vi "Main PC Station.vi"() -> ()   [LabVIEW 2014]
uses:
  ramki konfiguracyjne.ctl
  CANFrameControl.ctl
  klapki.ctl
  RaptorV_3/Users/K/Desktop/Nowe SbRio/PC/Queue message.ctl
  Program Files (x86)/National Instruments/LabVIEW 2014/examples/Design Patterns/Queued Message Handler/support/QMH Fundamentals - Message Cluster.ctl
  <vilib>/Utility/inputDevices.llb/closeJoystick.vi
  Global GPS.vi
  <vilib>/vision/driver/NI_Vision_Acquisition_Software.lvlib
  <vilib>/ptbypt/NI_PtbyPt.lvlib
panel:
  in  "Zresetuj monitor":bool
  in  "Przestarzała data":bool
  out "czas stopu":timestamp
  out "x-y":dbl
  in  "RESET STM":bool
  in  "STOP ??":bool
  out "timestamp last":timestamp
  out "Waveform Chart":cluster{dbl}(graph)
  in  "Boolean":bool
  out "tim 2":dbl format="%#.8g"
  out "output cluster 3":T1 {"seconds since 1Jan1904" format="%<%H:%M:%S\n%x>T"}
  in  "output cluster 2":T2 {"zadany" format="%<%H:%M:%S\n%x>T"}
  out "output cluster":T3 {"latitude (deg) 2" format="%#.8g"; "longitude (deg) 2" format="%#.8g"}
  out "Numeric 5":i32
  out "wyj pred":cluster{u16, u16, u16, u16, u16, u16} {"?" scale=0.0..65000.0; "?" scale=0.0..65000.0; "?" scale=0.0..65000.0; "?" scale=0.0..65000.0; "?" scale=0.0..65000.0; "?" scale=0.0..65000.0}
  in  "E-Stop":bool
  in  "zerowanie predkosci":T4[](array[typedef])=[{"identifier"=1, "extended?"=FALSE, "type"=0, "payload"=[1, 0, 0, 0, 0, 0, 0, 0]}, {"identifier"=2, "extended?"=FALSE, "type"=0, "payload"=[0, 0, 0, 0, 0, 0, 0]}] {"type" items=["CAN Data", "CAN Remote"]; "identifier" format="%.0x"}
  in  "hamulec 2":T4[](array[typedef])=[{"identifier"=1, "extended?"=FALSE, "type"=0, "payload"=[1, 0, 0, 0, 0, 0, 0, 0]}, {"identifier"=2, "extended?"=FALSE, "type"=0, "payload"=[0, 0, 0, 0, 0, 0, 0]}] {"type" items=["CAN Data", "CAN Remote"]; "identifier" format="%.0x"}
  out "axis info":T5
  out "Digital Waveform Graph":digitalwaveform(graph)
  out "wszystkie":T6(graph)
  out "UDP connection":bool
  in  "Tab Control 2":enum32{"CAN", "FPGA H&S", "SAFETY", "Kamera"}(tab)
  in  "Tab Control":T7(tab)
  in  "STM Prawy ID 2":u32=1
  in  "STM Lewy ID 1":u32=2
  in  "IDD 1":u8=1
  in  "IDD 2":u8=1
  in  "PRZOD L":T8={"Prąd"=10.0, "Kp"=4.0, "Ki"=1.2, "OK Button"=FALSE, "ID"=2, "IDD"=2} {"Ki" format="%.1f"; "Kp" format="%.1f"; "Prąd" format="%.1f"}
  in  "TYL L":T8={"Prąd"=10.0, "Kp"=4.0, "Ki"=1.2, "OK Button"=FALSE, "ID"=2, "IDD"=3} {"Ki" format="%.1f"; "Kp" format="%.1f"; "Prąd" format="%.1f"}
  in  "SRODEK L":T8={"Prąd"=10.0, "Kp"=4.0, "Ki"=1.2000000000000002, "OK Button"=FALSE, "ID"=2, "IDD"=4} {"Ki" format="%.1f"; "Kp" format="%.1f"; "Prąd" format="%.1f"}
  in  "SRODEK P":T8={"Prąd"=10.0, "Kp"=4.0, "Ki"=1.2000000000000002, "OK Button"=FALSE, "ID"=1, "IDD"=3} {"Ki" format="%.1f"; "Kp" format="%.1f"; "Prąd" format="%.1f"}
  in  "TYL P":T8={"Prąd"=10.0, "Kp"=4.0, "Ki"=1.2000000000000002, "OK Button"=FALSE, "ID"=1, "IDD"=4} {"Ki" format="%.1f"; "Kp" format="%.1f"; "Prąd" format="%.1f"}
  in  "PRZOD P":T8={"Prąd"=10.0, "Kp"=4.0000000000000036, "Ki"=1.2000000000000002, "OK Button"=FALSE, "ID"=1, "IDD"=2} {"Ki" format="%.1f"; "Kp" format="%.1f"; "Prąd" format="%.1f"}
  in  "wagi":T9={"l przod"=1.0, "l tyl"=1.0, "l srodek"=1.0, "p przod"=1.0, "p tyl"=1.0, "p srodek"=1.0} {"l przod" format="%#.6g"}
  in  "serwa i pompa":T10={"lewy tyl "=TRUE, "prawy tyl "=TRUE, "lewy przod "=TRUE, "środek"=TRUE, "prawy przod "=TRUE, "serwo 3"=TRUE, "serwo 4 "=TRUE, "przekaznik"=TRUE}
  in  "PWM4":T8={"Prąd"=0.0, "Kp"=4.0, "Ki"=1.2, "OK Button"=FALSE, "ID"=2, "IDD"=2} {"Ki" format="%.1f"; "Kp" format="%.1f"; "Prąd" format="%.1f"}
  in  "PWM5":T8={"Prąd"=0.0, "Kp"=4.0, "Ki"=1.2, "OK Button"=FALSE, "ID"=2, "IDD"=2} {"Ki" format="%.1f"; "Kp" format="%.1f"; "Prąd" format="%.1f"}
  in  "PWM6":T8={"Prąd"=0.0, "Kp"=4.0, "Ki"=1.2, "OK Button"=FALSE, "ID"=2, "IDD"=3} {"Ki" format="%.1f"; "Kp" format="%.1f"; "Prąd" format="%.1f"}
  in  "PWM7":T8={"Prąd"=0.0, "Kp"=4.0, "Ki"=1.2000000000000002, "OK Button"=FALSE, "ID"=2, "IDD"=4} {"Ki" format="%.1f"; "Kp" format="%.1f"; "Prąd" format="%.1f"}
  in  "PWM2":T8={"Prąd"=0.0, "Kp"=4.0, "Ki"=1.2000000000000002, "OK Button"=FALSE, "ID"=1, "IDD"=3} {"Ki" format="%.1f"; "Kp" format="%.1f"; "Prąd" format="%.1f"}
  in  "PWM3":T8={"Prąd"=0.0, "Kp"=4.0, "Ki"=1.2000000000000002, "OK Button"=FALSE, "ID"=1, "IDD"=4} {"Ki" format="%.1f"; "Kp" format="%.1f"; "Prąd" format="%.1f"}
  in  "PWM1":T8={"Prąd"=0.0, "Kp"=4.0000000000000036, "Ki"=1.2000000000000002, "OK Button"=FALSE, "ID"=1, "IDD"=2} {"Ki" format="%.1f"; "Kp" format="%.1f"; "Prąd" format="%.1f"}
  in  "MANIPULATOR ID 3":u32=3
  in  "SERWO 6":u8(slide)=127 scale=0.0..255.0
  in  "SERWO 5":u8(slide)=127 scale=0.0..255.0
  in  "SERWO 4":u8(slide)=127 scale=0.0..255.0
  in  "SERWO 3":u8(slide)=127 scale=0.0..255.0
  in  "Stop głębokość":bool
  in  "Stop wózek":bool
  in  "Wiertło PWM":u8(slide)=128 scale=0.0..255.0
  in  "Wózek PWM":u8(slide)=128 scale=0.0..255.0
  in  "Głębokość PWM":u8(slide)=128 caption="Vertical Pointer Slide" scale=0.0..255.0
  in  "ON/OFF Wiertło":bool
  in  "speed głębokość":u8
  in  "speed wózek":u8
  out "krańcówka 4":bool
  out "krańcówka 3":bool
  out "krańcówka 2":bool
  out "krańcówka":bool
  in  "PROBNK ID 4":u32=3
  in  "Wózek up":bool
  in  "Głębokość down":bool
  in  "Głębokość up":bool
  in  "Wózek down":bool
  out "glebokosc aktualna":dbl(slide) scale=-150.0..220.0
  out "PH":u16(knob) scale=0.0..4095.0
  out "wilgotność i temperatura":string
  out "Środek P":cluster{"mean":dbl, u16}(graph)
  out "PRZOD L":cluster{"mean":dbl, u16}(graph)
  out "TYL L":cluster{"mean":dbl, u16}(graph)
  out "SRODEK L":cluster{"mean":dbl, u16}(graph)
  out "przod P":cluster{"mean":dbl, u16}(graph)
  out "Tyl P":cluster{"mean":dbl, u16}(graph)
  out "Frames":string[][](table)
  in  "Hexadecimal?":bool
  in  "Widocznosc ramek":bool=TRUE
  out "okres 100[ms]":dbl format="%.3g"
  out "ilosc mesagy":dbl
  in  "okres watchdoga":u32=100
  in  "wlacz watchdoga":bool
  out "temperatura":sgl(slide) scale=25.0..70.0
  in  "Total (%)":dbl(knob) scale=0.0..100.0
  in  "System Reset":bool
  out "kolejka odbior":i32
  out "kolejka wysylanie":i32
  in  "stop UDP 2":bool
  in  "udp to sbrio  2":bool
  in  "eventy stop":bool
  out "send ind":i32
  in  "stop queue":bool
  out "receive ind":i32
  in  "UDP odbior in":bool
  in  "stop all":bool
  in  "UDP from sb 2":bool
  in  "UDP to sb 2":bool
  out "eventy ind":i32
  out "Numeric 3":i32
  out "Numeric 4":i32
  out "Image":T11(plugin-control)
  in  "Camera Name":refnum<k21> caption="IMAQdx Session"
  in  "ON/OFF CAM":bool
  out "Acquiring":bool
  in  "Stop 2":bool
  out "Buffer Number 3":u32
  in  "stop UDP":bool
  in  "UDP from sb":bool
  in  "UDP to sb":bool
  out "brak polaczenia":bool
  out "Numeric 2":i32
  out "Numeric":i32
  out "połączenie RT":bool
  out "button 4":bool
  out "button 3":bool
  out "button 2":bool
  out "button 1":bool
  in  "index joya jazda":i32
  in  "device index":i32=4
  out "zakres X":bool
  out "wysylanie":bool
  out "blokadaa":bool
  out "zakres Y":bool
  in  "Sterowanie w ukladzie narzędzia":bool
  out "graph 2":cluster{i32[], i32[]}[](graph)
  out "String wysylany":string
  out "Pz":dbl(slide) scale=0.0..1149.0
  out "Py":dbl(slide) scale=0.0..1075.0
  out "Px":dbl(slide) scale=0.0..1075.0
  out "q5":dbl format="%.2f"
  out "q4":dbl format="%.2f"
  out "q3":dbl format="%.2f"
  out "q2":dbl format="%.2f"
  out "q1":dbl format="%.2f"
  in  "Strin wysłany":string
  out "pwm 1":dbl
  out "pwm 2":dbl
  out "pwm 3":dbl
  out "pwm 4":dbl
  out "pwm 5":dbl
  out "pwm 6":dbl
  out "pwm 7":dbl
  out "zakres Z":bool
  out "cluster manipulator":T12
  in  "UDP odbior":bool
  out "cluster jazda":T13
  out "zak1":bool
  out "zak2":bool
  out "Blokada jazda":bool
  in  "udp to sbrio":bool
  out "hamowanie":bool
  out "hamowaniejazda":dbl
  out "obrotjazda":dbl
  out "skretjazda":dbl
  out "pwmjazda":dbl
  out "obrot":string
  out "skret":string
  out "pwm":string
  out "graph 1":cluster{i32[], i32[]}[](graph)
  out "hamowanie string":string
  out "obrot string":string
  in  "max obrót":dbl(slide) caption="max obrot" scale=0.0..1.0
  in  "max pwm skrecanie":dbl(slide)=1.0 scale=0.0..1.0
  in  "max pwm przod":dbl(slide)=1.0 min=0.0 max=255.0 scale=0.0..1.0
  out "Wysylanie jazda":bool
  out "wyslany":string
  out "jazda":string
  # "STARE"
  # "T-"
  # "T+"
  # "gimbal 1"
  # "gimbal 2"
  # "pochyl chwytak"
  # "PWM 3 os Y\nPWM 4 os X\nPWM 5 T"
  # "chwytak O/Z"
  # "obrot chwytak"
  # "ramie 1"
  # "PWM1 os X \nPWM2 os Y\nPWM 6 T"
  # "ramie 2"
  # "obrot podstawa"
  # "Os Y+"
  # "PWM 7 T"
  # "Os X +"
  # "AKTUALNE"
  # "WYSYLANE"
  # "WYSYLANIE"
  # "- max skrecanie +"
  # "- max jazda +"
  # "hamowanie"
  # "sam OBROT"
  # "- max obrot +"
  # "OBROT"
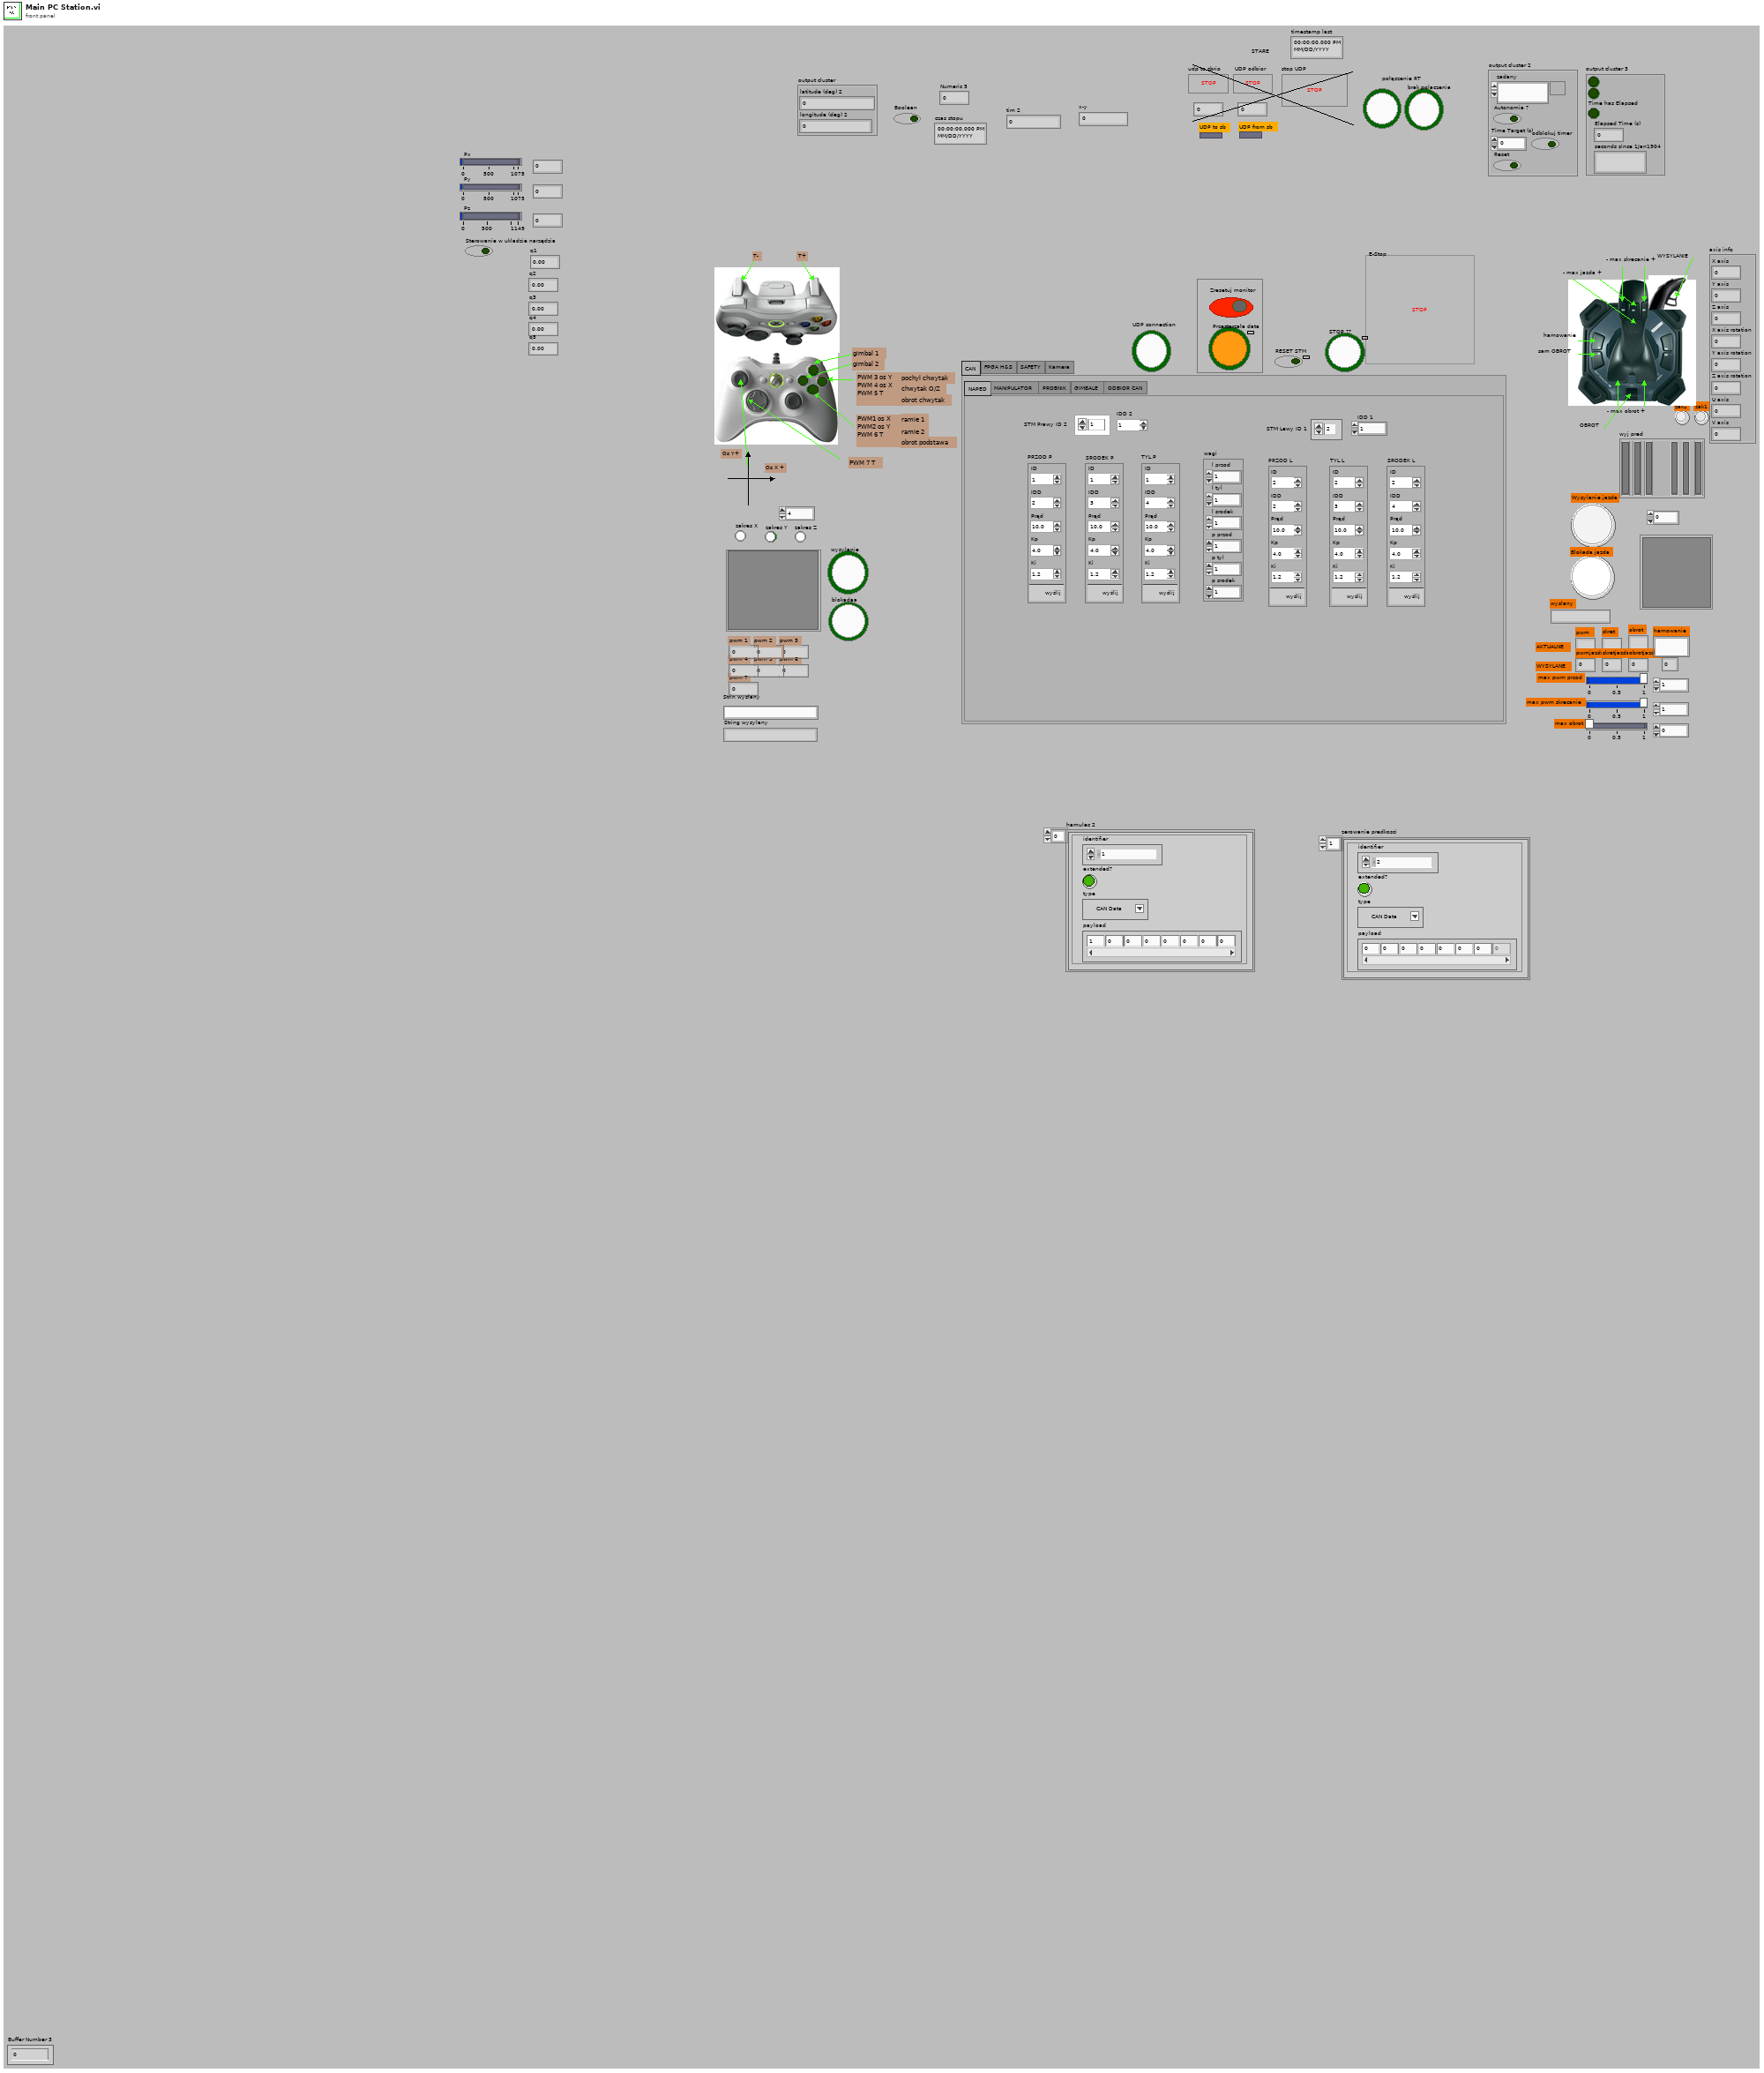
[diagram p1: front panel]
types:
  T1 = cluster{bool, bool, "Time has Elapsed":bool, "Elapsed Time (s)":dbl, "seconds since 1Jan1904":timestamp}
  T2 = cluster{"zadany":timestamp, "Autonomia ?":bool, "Time Target (s)":dbl, "Reset":bool, "odblokuj timer":bool}
  T3 = cluster{"latitude (deg) 2":dbl, "longitude (deg) 2":dbl}
  T4 = typedef "CANFrameControl.ctl" = cluster{"identifier":u32, "extended?":bool, "type":u8, "payload":u8[]}
  T5 = cluster{"X axis":i32, "Y axis":i32, "Z axis":i32, "X axis rotation":i32, "Y axis rotation":i32, "Z axis rotation":i32, "U axis":i32, "V axis":i32}
  T6 = cluster{"mean":dbl, "mean":dbl, "mean":dbl, "mean":dbl, "mean":dbl, "mean":dbl}
  T7 = enum32{"NAPED", "MANIPULATOR", "PROBNIK", "GIMBALE", "ODBIOR CAN"}
  T8 = typedef "ramki konfiguracyjne.ctl" = cluster{"Prąd":dbl, "Kp":dbl, "Ki":dbl, "OK Button":bool, "ID":u32, "IDD":u8}
  T9 = cluster{"l przod":dbl, "l tyl":dbl, "l srodek":dbl, "p przod":dbl, "p tyl":dbl, "p srodek":dbl}
  T10 = typedef "klapki.ctl" = cluster{"lewy tyl ":bool, "prawy tyl ":bool, "lewy przod ":bool, "środek":bool, "prawy przod ":bool, "serwo 3":bool, "serwo 4 ":bool, "przekaznik":bool}
  T11 = typedef "IMAQ Image.ctl" = refnum<image>
  T12 = cluster{"pwm 1":dbl, "pwm 2":dbl, "pwm 3":dbl, "pwm 4":dbl, "pwm 5":dbl, "pwm 6":dbl, "pwm 7":dbl}
  T13 = cluster{"pwmjazda":dbl, "skretjazda":dbl, "obrotjazda":dbl, "hamowaniejazda":dbl}
  T14 = typedef "QMH Fundamentals - Message Cluster.ctl" = cluster{"Message":string, "Message Data":variant}
  T15 = typedef "Queue message.ctl" = cluster{"Message":string, "Message Data":variant}
  T16 = enum16{"Rising Edge", "Falling Edge", "Any Edge"}
  T17 = typedef "Wyjscia joya.ctl" = cluster{"button 1":bool, "button 2":bool, "button 3":bool, "button 4":bool, "button 5":bool, "button 6":bool, "button 7":bool, "button 8":bool, "button 9":bool, "POV":bool, "button 10":bool}
  T18 = cluster{"STM Lewy ID 1":u32, "STM Prawy ID 2":u32, "IDD 1":u8, "IDD 2":u8}
  T19 = cluster{"remote port":u16, u32, "port":refnum<k16>, "error out":errorcluster}
  T20 = cluster{"cluster_jazda":cluster{"pwmjazda":dbl, "skretjazda":dbl, "obrotjazda":dbl, "hamowaniejazda":dbl}, "cluster_manipulator":cluster{"pwm 1":dbl, "pwm 2":dbl, "pwm 3":dbl, "pwm 4":dbl, "pwm 5":dbl, "pwm 6":dbl, "pwm 7":dbl}, "GIMBALE":cluster{"Gimbal 1":cluster{"OSY":dbl, "OSY X":dbl}, "Gimbal 2":cluster{"OSY":dbl, "OSY X":dbl}}}
  T21 = cluster{"button 1":bool, "button 2":bool, "button 3":bool, "button 4":bool, "button 5":bool}
  T22 = typedef "IMAQdx.ctl" = refnum<k21>
  T23 = cluster{"SERWO 6":u8, "SERWO 5":u8, "SERWO 4":u8, "SERWO 3":u8, "ON/OFF Wiertło":bool, "Wiertło PWM":u8, "Wózek PWM":u8, "Stop głębokość":bool, "Głębokość PWM":u8, "speed wózek":u8, "Wózek up":bool, "Wózek down":bool, "Stop wózek":bool, "PROBNK ID 4":u32}
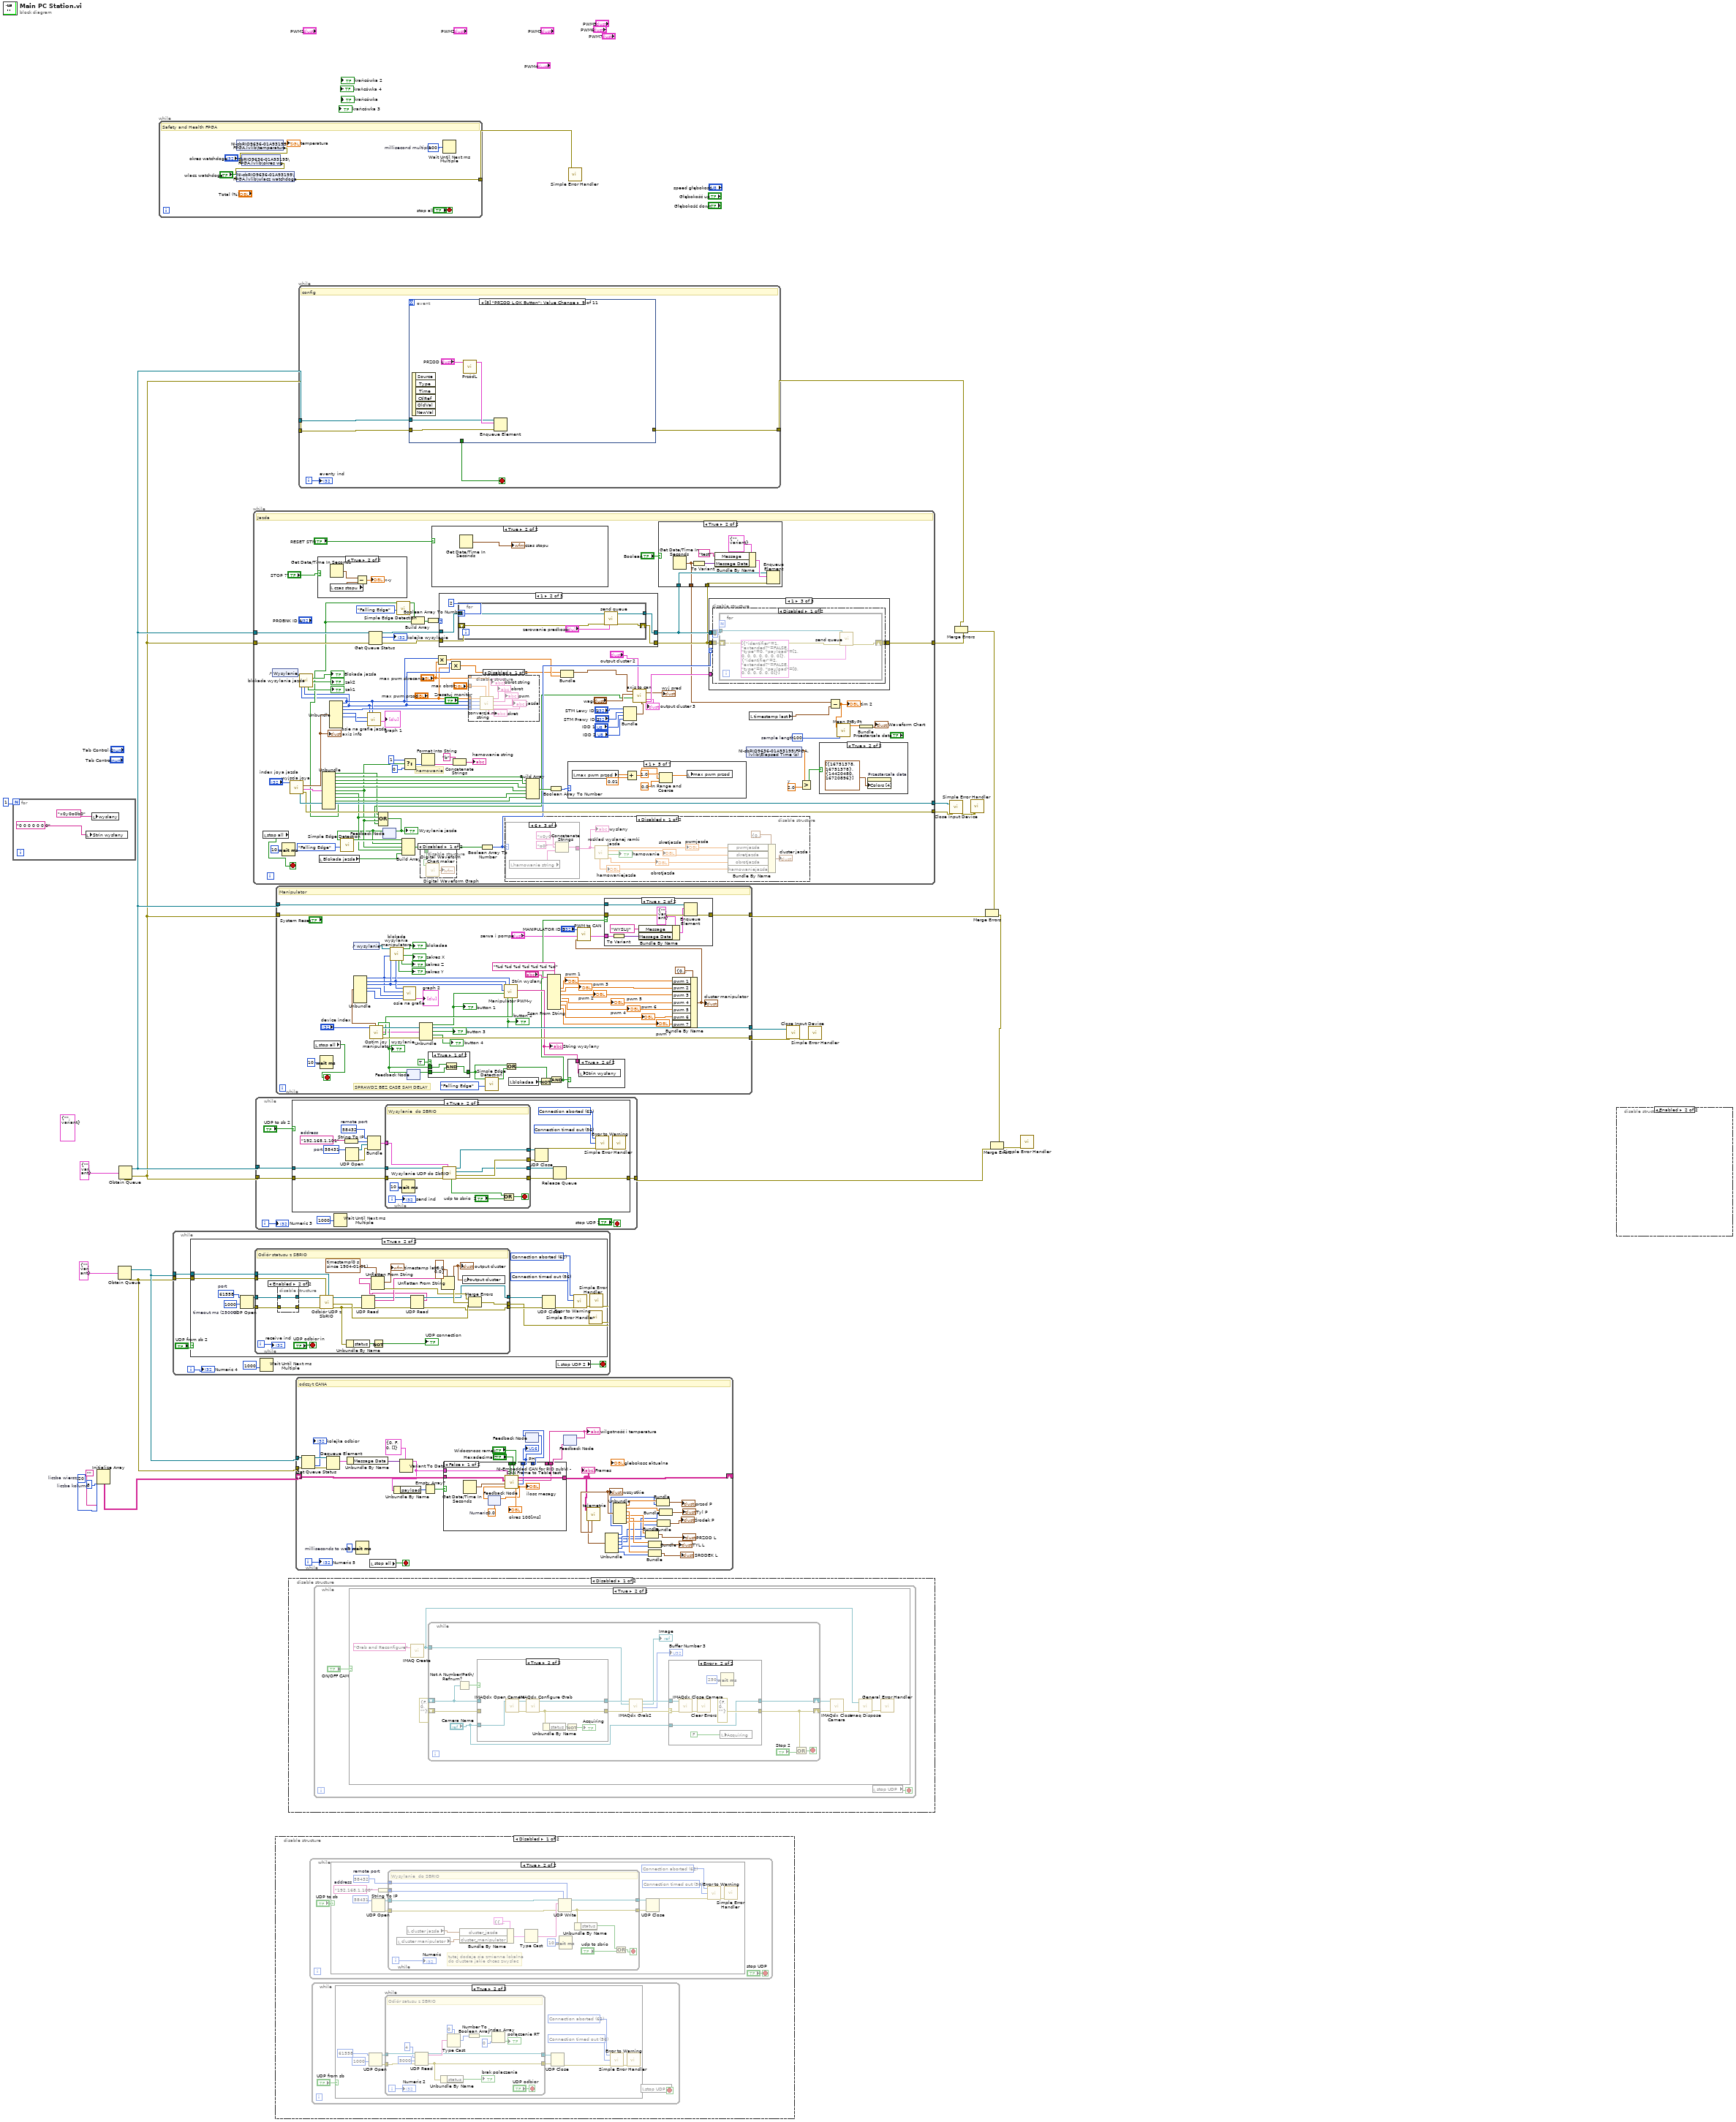
[diagram p0: block diagram]
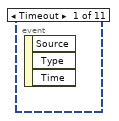
[diagram p7: hidden frame]
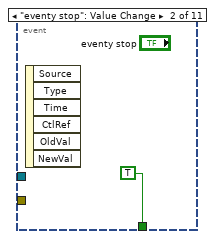
[diagram p8: hidden frame]
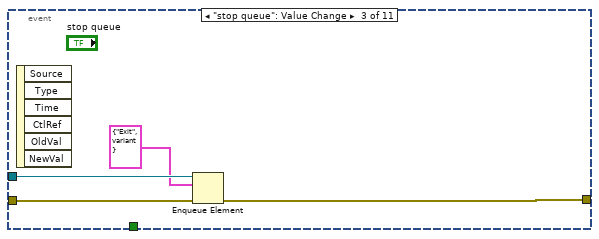
[diagram p9: hidden frame]
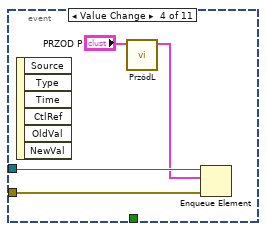
[diagram p10: hidden frame]
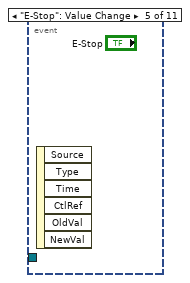
[diagram p11: hidden frame]
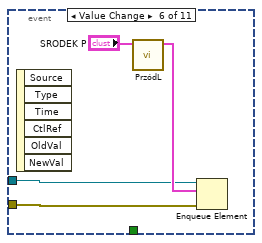
[diagram p12: hidden frame]
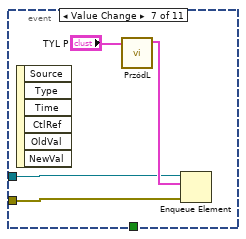
[diagram p13: hidden frame]
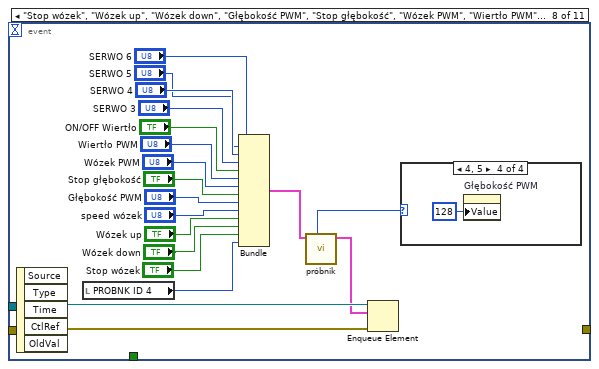
[diagram p14: hidden frame]
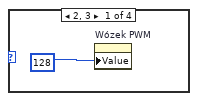
[diagram p15: hidden frame]
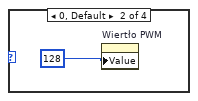
[diagram p16: hidden frame]
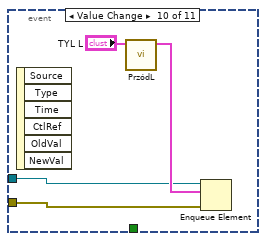
[diagram p18: hidden frame]
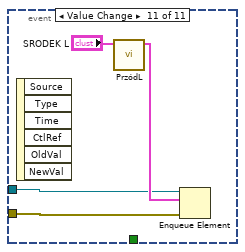
[diagram p19: hidden frame]
diagram:
  w8 = 20  # liczba wierszy
  w7 = 5  # liczba kolumn
  (unwired) T15 {"Message"="", "Message Data"=variant} ("Message Cluster")
  n1 = for {
    N: 1 -> [_]
    n2 = local write "Strin wysłany"("0 0 0 0 0 0 0") -> ()
    n3 = local write "wyslany"("x0y0o0b0") -> ()
  }
  n4 = Initialize Array("" ("Empty String Constant"), w8, w7) -> (w5:string[][])
  n5 = Obtain Queue(element data type=T14 {"Message"="", "Message Data"=variant} ("Message Cluster")) -> (queue out=w3:refnum<queue>, error out=w2:errorcluster)  [unwired: 4 in, 1 out]
  n6 = Obtain Queue(element data type=T14 {"Message"="", "Message Data"=variant} ("Message Cluster")) -> (queue out=w13:refnum<queue>, error out=w12:errorcluster)  [unwired: 4 in, 1 out]
  n7 = while {
    tunnel: [w30] -> w1
    stop <- "stop all" stop-if-true
    w34 = u32 100  # millisecond multiple
    # "Safety and Health FPGA"
    n8 = shared-variable "NI-sbRIO9636-01A93195\\FPGA.lvlib\\temperatura"() -> (→"temperatura":sgl, error out=w29:errorcluster)  [unwired: 1 in]
    n9 = shared-variable "NI-sbRIO9636-01A93195\\FPGA.lvlib\\okres wg"("okres watchdoga", error in=w29) -> (error out=w31:errorcluster)
    n10 = shared-variable "NI-sbRIO9636-01A93195\\FPGA.lvlib\\wlacz watchdoga"("wlacz watchdoga", error in=w31) -> (error out=w30:errorcluster)
    n11 = Wait Until Next ms Multiple(millisecond multiple=w34) -> ()  [unwired: 1 out]
  }
  n12 = while {
    tunnel: w3 -> [w37]
    tunnel: w2 -> [w36]
    i -> [w39]
    stop <- w40 stop-if-true
    n13 = case shown="True" "UDP from sb 2" {
      tunnel: w37 -> [_ w44]
      tunnel: w36 -> [_ w43]
      frame False {
      }
      frame True {
        w53 = 1000  # timeout ms (25000)
        w50 = 56 items=["No Error", "Argument Error", "Memory Full", "Out of Zone", "End of File", "File Already Open", "Generic File IO Error", "File Not Found", "File Permission Error", "Disk Full", "Duplicate Path", "Too Many Files Open", "Not Enabled", "Resource File Not Found", "Cannot Add Resource", "Resource Not Found", "Image Not Found", "Image Memory Error", "Pen Does Not Exist", "Config Bad Type", "Config Token Not Found", "Config Parse Error", "Config Memory Error", "Bad External Code Format", "Bad External Code Offset", "External Code Not Present", "Null Window", "Destroy Window Mixup", "Null Menu", "Print Aborted", "Bad Print Record", "Print Driver Error", "Windows Error During Print", "Memory Error During Print", "Print Dialog Error", "Generic Print Error", "Invalid Device Refnum", "Device Not Found", "Device Parameter Error", "Device Unit Error", "Can't Open Device", "Device Call Aborted", "Generic Error", "Cancelled By User", "Object ID Too Low", "Object ID Too High", "Object Not In Heap", "Unknown Heap", "Bad DefProc ID", "DefProc Not In Table", "Message Out Of Range", "Null Method", "Unknown Message", "Manager Call Not Supported", "Bad address", "Connection In progress", "Connection timed out", "Connection is already in progress", "Network attribute not supported", "Network error", "Address in use", "System out of memory", "Connection aborted", "Connection refused", "Connection is not connected", "Connection is already connected", "Connection closed", "Initialize error (interapplication manager)", "Bad occurrence", "Wait on unbound occurrence handler", "Occurrence queue overflow", "Bad path", "Semaphore not signaled", "Unrecognized type (interapplication manager)"] ("3rd Error to Convert")
        w51 = 62 items=["No Error", "Argument Error", "Memory Full", "Out of Zone", "End of File", "File Already Open", "Generic File IO Error", "File Not Found", "File Permission Error", "Disk Full", "Duplicate Path", "Too Many Files Open", "Not Enabled", "Resource File Not Found", "Cannot Add Resource", "Resource Not Found", "Image Not Found", "Image Memory Error", "Pen Does Not Exist", "Config Bad Type", "Config Token Not Found", "Config Parse Error", "Config Memory Error", "Bad External Code Format", "Bad External Code Offset", "External Code Not Present", "Null Window", "Destroy Window Mixup", "Null Menu", "Print Aborted", "Bad Print Record", "Print Driver Error", "Windows Error During Print", "Memory Error During Print", "Print Dialog Error", "Generic Print Error", "Invalid Device Refnum", "Device Not Found", "Device Parameter Error", "Device Unit Error", "Can't Open Device", "Device Call Aborted", "Generic Error", "Cancelled By User", "Object ID Too Low", "Object ID Too High", "Object Not In Heap", "Unknown Heap", "Bad DefProc ID", "DefProc Not In Table", "Message Out Of Range", "Null Method", "Unknown Message", "Manager Call Not Supported", "Bad address", "Connection In progress", "Connection timed out", "Connection is already in progress", "Network attribute not supported", "Network error", "Address in use", "System out of memory", "Connection aborted", "Connection refused", "Connection is not connected", "Connection is already connected", "Connection closed", "Initialize error (interapplication manager)", "Bad occurrence", "Wait on unbound occurrence handler", "Occurrence queue overflow", "Bad path", "Semaphore not signaled", "Unrecognized type (interapplication manager)"] ("1st Error to Convert")
        w45 = u16 61558  # port
        n14 = UDP Open(9:w53, 11:w45) -> (port=w46:refnum<k16>, 0:w47:errorcluster)  [unwired: 3 in, 1 out]
        n15 = while {
          tunnel: w46 -> [w64]
          tunnel: w47 -> [w65]
          tunnel: [w56] -> w48
          tunnel: [w59] -> w54
          tunnel: [w71] -> w42
          tunnel: w44 -> [w76]
          tunnel: w43 -> [w75]
          i -> [w78]
          stop <- "UDP odbior in" stop-if-true
          # "Odiór statusu z SBRIO"
          n16 = disable-structure shown="Enabled" {
            disable-tunnel: w65 -> [w84 w85]
            disable-tunnel: w64 -> [w83 w86]
            disable-tunnel: [w82 w86] -> w63
            disable-tunnel: [w81 w85] -> w62
            frame Disabled {
              n17 = UDP Read(connection ID=w83, 8:w84) -> (error out=w81:errorcluster, 3:w82:refnum<k16>)  [unwired: 2 in, 3 out]
            }
            frame Enabled {
            }
          }
          n18 = call "Odbiór UDP z SbRIO.vi"("Queue in"=w76, "error in queue"=w75, "error in udp (no error)"=w62, "port"=w63) -> ("error out udp"=w69:errorcluster, "error out variant"=w72:errorcluster, "UDP Network Connection out"=w67:refnum<k16>)  [unwired: 5 in]
          n19 = Unbundle By Name(w69) -> ("status"=w79:bool)
          n20 = UDP Read(connection ID=w67, 8:w69) -> (data out=w66:string, error out=w58:errorcluster, 3:w57:refnum<k16>)  [unwired: 2 in, 2 out]
          n21 = Not(x=w79) -> (.not. x?=→"UDP connection":bool)
          n22 = UDP Read(connection ID=w57, 8:w58) -> (data out=w55:string, error out=w59:errorcluster, 3:w56:refnum<k16>)  [unwired: 2 in, 2 out]
          n23 = Unflatten From String(type=timestamp(0 s since 1904-01-01) ("seconds since 1Jan1904"), binary string=w55) -> (value=→"timestamp last":timestamp, error out=w68:errorcluster)  [unwired: 3 in, 1 out]
          n24 = Unflatten From String(type=T3 {"latitude (deg) 2"=0.0, "longitude (deg) 2"=0.0} ("output cluster"), binary string=w66) -> (value=w70:T3, error out=w73:errorcluster)  [unwired: 3 in, 1 out]
          "output cluster" <- w70
          n25 = global write "Global GPS.vi" "output cluster"(w70) -> ()
          n26 = Merge Errors(w68, w73, w72) -> (w71:errorcluster)
          "receive ind" <- w78
        }
        n27 = UDP Close(connection ID=w48, 8:w54) -> (error out=w52:errorcluster)  [unwired: 1 out]
        n28 = call <vilib>:"Error to Warning.vi"("1st Error to Convert"=w51, "3rd Error to Convert"=w50, "error in"=w52) -> ("warning out"=w49:errorcluster)  [unwired: 3 in, 9 out]
        n29 = call <vilib>:"Simple Error Handler.vi"("error in (no error)"=w42) -> ()  [unwired: 1 in, 8 out]
        n30 = call <vilib>:"Simple Error Handler.vi"("error in (no error)"=w49) -> ()  [unwired: 1 in, 8 out]
      }
    }
    n31 = Wait Until Next ms Multiple(millisecond multiple=u32 1000 ("milliseconds to wait")) -> ()  [unwired: 1 out]
    n32 = local read "stop UDP 2"() -> (w40:bool)
    "Numeric 4" <- w39
  }
  n33 = while {
    tunnel: [w155] -> w24
    tunnel: [w154] -> w23
    tunnel: w13 -> [w134]
    tunnel: w12 -> [w135]
    tunnel: [w136] -> w14
    stop <- w127 stop-if-true
    w89 = 2.0  # y
    w93 = 100  # sample length
    # "hamowanie"
    # "Jazda"
    n34 = local read "stop all"() -> (w127:bool)
    n35 = control-ref of="Wysylanie jazda"() -> (w167:refnum<vi>)
    n36 = Wait (ms)(milliseconds to wait=u32 10) -> ()  [unwired: 1 out]
    n37 = call "wyjscia joya.vi"("index joya jazda"="index joya jazda") -> ("error out"=w154:errorcluster, "wyjscia joya"=w153:T17, "axis info"=w124:T5, "Refnum out"=w155:refnum<k1>)  [unwired: 5 in]
    "axis info" <- w124
    n38 = case shown="True" "STOP ??" {
      frame False {
      }
      frame True {
        n39 = Get Date/Time In Seconds() -> (seconds since 1Jan1904=w172:timestamp)
        n40 = local read "czas stopu"() -> (w171:timestamp)
        n41 = Subtract(x=w172, y=w171) -> (x-y=→"x-y":dbl)
      }
    }
    n42 = local read "Blokada jazda"() -> (w168:bool)
    n43 = Unbundle(w153) -> ("button 1"=w146:bool, "button 2"=w152:bool, "button 3"=w151:bool, "button 4"=w150:bool, "button 5"=w149:bool, "button 6"=w144:bool, "button 7"=w145:bool, "button 8"=w148:bool, "button 9"=w147:bool, "POV"=w121:bool)  [unwired: 1 out]
    n44 = Unbundle(w124) -> ("X axis"=w110:i32, "Y axis"=w107:i32, "Z axis"=w138:i32, "X axis rotation"=w139:i32, "Y axis rotation"=w140:i32)  [unwired: 3 out]
    n45 = call "blokada wysylania jazda.vi"("Y axis"=w107, "X axis"=w110, "Boolean in"=w167) -> ("zak2"=→"zak2":bool, "blokada jazdy"=→"Blokada jazda":bool, "zak1"=→"zak1":bool)  [unwired: 6 in]
    n46 = call "osie na grafie jazda.vi"("Y axis rotation"=w140, "X axis rotation"=w139, "Y axis"=w107, "X axis"=w110) -> ("graph 1"=→"graph 1":cluster{i32[], i32[]}[])  [unwired: 7 in]
    n47 = Get Queue Status(queue=w134, error in (no error)=w135) -> (queue out=w126:refnum<queue>, error out=w125:errorcluster, # elements in queue=→"kolejka wysylanie":i32)  [unwired: 1 in, 5 out]
    n48 = feedback #1() -> (w130:bool)  [unwired: 1 in]
    n49 = call "Simple Edge Detection.vi"("Mode"=T16."Falling Edge", "clk_in"=w130) -> ("edge?"=w157:bool)  [unwired: 9 in]
    n50 = call "Simple Edge Detection.vi"("Mode"=T16."Falling Edge", "clk_in"=w121) -> ("edge?"=w122:bool)  [unwired: 9 in]
    n51 = Build Array(w157, w130, w144, w145, w168) -> (w129:bool[])
    n52 = Select(t=1, s=w144, f=0) -> (s? t:f=w143:i32)
    n53 = Build Array(w122, w121) -> (w120:bool[])
    n54 = disable-structure shown="Disabled" {
      disable-tunnel: w129 -> [w233 _]
      frame Disabled {
        n55 = call "Digital Waveform Chart maker.vi"("Array"=w233) -> ("digital waveform"=→"Digital Waveform Graph":digitalwaveform)  [unwired: 3 in]
      }
      frame Enabled {
      }
    }
    n56 = Format Into String(w143) -> (resulting string=w161:string)  [unwired: 3 in, 1 out]
    n57 = Boolean Array To Number(Boolean array=w120) -> (number=w119:u32)
    n58 = case shown="True" "RESET STM" {
      frame False {
      }
      frame True {
        n59 = Get Date/Time In Seconds() -> (seconds since 1Jan1904=→"czas stopu":timestamp)
      }
    }
    n60 = Multiply(x=w110, y="max pwm skrecanie") -> (x*y=w109:dbl)
    n61 = case shown="1" w119 {
      tunnel: [w216 w218 w228] -> w100
      tunnel: w126 -> [w216 w221 w229]
      tunnel: w125 -> [w215 w220 w230]
      tunnel: [w215 w219 w231] -> w99
      frame 0, Default {
      }
      frame 1 {
        n62 = for {
          N: 2 -> [_]
          tunnel: w221 -> [w226]
          shift-right: [w224] -> w219
          shift-left: w220 -> [w225]
          tunnel: [w222] -> w218
          n63 = call "send queue.vi"("zerowanie predkosci"="zerowanie predkosci", "error in (no error)"=w225, "Queue in"=w226) -> ("error out"=w224:errorcluster, "queue out"=w222:refnum<queue>)  [unwired: 7 in]
        }
      }
      frame 2 {
        n64 = call "send queue.vi"("zerowanie predkosci"="hamulec 2", "error in (no error)"=w230, "Queue in"=w229) -> ("error out"=w231:errorcluster, "queue out"=w228:refnum<queue>)  [unwired: 7 in]
      }
    }
    n65 = Multiply(x=w107, y="max pwm przod") -> (x*y=w108:dbl)
    n66 = Concatenate Strings("b", w161) -> (→"hamowanie string":string)
    n67 = disable-structure shown="Disabled" {
      disable-tunnel: w138 -> [w192 _]
      disable-tunnel: w107 -> [w191 _]
      disable-tunnel: w110 -> [w190 _]
      disable-tunnel: "max obrót" -> [w188 _]
      disable-tunnel: "max pwm przod" -> [w184 _]
      disable-tunnel: "max pwm skrecanie" -> [w182 _]
      frame Disabled {
        n68 = call "conversja na string.vi"("max pwm skrecanie"=w182, "max obrót"=w188, "Z axis"=w192, "Y axis"=w191, "X axis"=w190, "max pwm przod"=w184) -> ("String 5"=→"jazda":string, "String 3"=→"pwm":string, "String 2"=→"obrot":string, "String 4"=→"obrot string":string, "String"=→"skret":string)  [unwired: 1 in]
      }
      frame Enabled {
      }
    }
    n69 = Boolean Array To Number(Boolean array=w129) -> (number=w128:u32)
    n70 = disable-structure shown="Disabled" {
      disable-tunnel: w128 -> [w193 _]
      frame Disabled {
        n71 = case shown="6" w193 {
          tunnel: ["x0y0o0b0" w205 w209 w214] -> w198
          frame 1, Default {
          }
          frame 2 {
            n72 = local read "jazda"() -> (w206:string)
            n73 = Concatenate Strings(w206, "o0", "b0") -> (w205:string)
          }
          frame 6 {
            n74 = local read "hamowanie string"() -> (w207:string)
            n75 = Concatenate Strings("x0y0", "o0", w207) -> (w209:string)
          }
          frame 10 {
            n76 = local read "obrot string"() -> (w212:string)
            n77 = Concatenate Strings("x0y0", w212, "b0") -> (w214:string)
          }
        }
        "wyslany" <- w198
        n78 = call "rozklad wyslanej ramki jazda.vi"("Wyslany"=w198) -> ("obrotjazda"=w196:dbl, "hamowanie"=→"hamowanie":bool, "skretjazda"=w195:dbl, "pwmjazda"=w194:dbl, "hamowaniejazda"=w197:dbl)  [unwired: 6 in]
        "pwmjazda" <- w194
        "skretjazda" <- w195
        "obrotjazda" <- w196
        "hamowaniejazda" <- w197
        n79 = Bundle By Name(cluster=T13 {"pwmjazda"=0.0, "skretjazda"=0.0, "obrotjazda"=0.0, "hamowaniejazda"=0.0} ("output cluster"), "pwmjazda"=w194, "skretjazda"=w195, "obrotjazda"=w196, "hamowaniejazda"=w197) -> (→"cluster jazda":T13)
      }
      frame Enabled {
      }
    }
    n80 = Build Array(w151, w152, w150, w149, w148, w147) -> (w159:bool[])
    n81 = Boolean Array To Number(Boolean array=w159) -> (number=w158:u32)
    n82 = Bundle(w108, w109) -> (w104:cluster{dbl, dbl})  [unwired: 1 in]
    n83 = case shown="1" w158 {
      frame 8 {
        n84 = local read "max pwm skrecanie"() -> (w259:dbl)
        n85 = Add(x=w259, y=0.01) -> (x+y=w255:dbl)
        n86 = In Range and Coerce(upper limit=1.0, x=w255, lower limit=0.0) -> (coerced(x)=w254:dbl)  [unwired: 1 out]
        n87 = local write "max pwm skrecanie"(w254) -> ()
      }
      frame 16 {
        n88 = local read "max obrót"() -> (w265:dbl)
        n89 = Subtract(x=w265, y=0.01) -> (x-y=w260:dbl)
        n90 = In Range and Coerce(upper limit=1.0, x=w260, lower limit=0.0) -> (coerced(x)=w261:dbl)  [unwired: 1 out]
        n91 = local write "max obrót"(w261) -> ()
      }
      frame 32 {
        n92 = local read "max obrót"() -> (w271:dbl)
        n93 = Add(x=w271, y=0.01) -> (x+y=w266:dbl)
        n94 = In Range and Coerce(upper limit=1.0, x=w266, lower limit=0.0) -> (coerced(x)=w267:dbl)  [unwired: 1 out]
        n95 = local write "max obrót"(w267) -> ()
      }
      frame 0, Default {
      }
      frame 1 {
        n96 = local read "max pwm przod"() -> (w272:dbl)
        n97 = Add(x=w272, y=0.01) -> (x+y=w273:dbl)
        n98 = In Range and Coerce(upper limit=1.0, x=w273, lower limit=0.0) -> (coerced(x)=w274:dbl)  [unwired: 1 out]
        n99 = local write "max pwm przod"(w274) -> ()
      }
      frame 2 {
        n100 = local read "max pwm przod"() -> (w278:dbl)
        n101 = Subtract(x=w278, y=0.01) -> (x-y=w279:dbl)
        n102 = In Range and Coerce(upper limit=1.0, x=w279, lower limit=0.0) -> (coerced(x)=w280:dbl)  [unwired: 1 out]
        n103 = local write "max pwm przod"(w280) -> ()
      }
      frame 4 {
        n104 = local read "max pwm skrecanie"() -> (w289:dbl)
        n105 = Subtract(x=w289, y=0.01) -> (x-y=w286:dbl)
        n106 = In Range and Coerce(upper limit=1.0, x=w286, lower limit=0.0) -> (coerced(x)=w287:dbl)  [unwired: 1 out]
        n107 = local write "max pwm skrecanie"(w287) -> ()
      }
    }
    n108 = Bundle("STM Lewy ID 1"="STM Lewy ID 1", "STM Prawy ID 2"="STM Prawy ID 2", "IDD 1"="IDD 1", "IDD 2"="IDD 2") -> (w114:T18)  [unwired: 1 in]
    n109 = call "axis to can.vi"("wej  ID"=w114, "output cluster 3"="output cluster 2", "wej wagi"="wagi", "wej ster"=w104) -> ("array of cans"=w132:T4[], "wyj pred"=→"wyj pred":cluster{u16, u16, u16, u16, u16, u16}, "output cluster 2"=→"output cluster 3":T1, "wyślij"=w101:bool)  [unwired: 1 in, 3 out]
    n110 = Compound Arithmetic op=OR(w146, w145, w144, w101) -> (w131:bool)
    "Wysylanie jazda" <- w131
    n111 = feedback-in #1(w131) -> ()
    n112 = case shown="True" "Boolean" {
      tunnel: w100 -> [_ w177]
      tunnel: w99 -> [_ w176]
      tunnel: [_ w175] -> w97
      frame False {
      }
      frame True {
        n113 = Get Date/Time In Seconds() -> (seconds since 1Jan1904=w175:timestamp)
        n114 = To Variant(anything=w175) -> (Variant=w179:variant)
        n115 = Bundle By Name(cluster=T14 {"Message"="", "Message Data"=variant} ("Message Cluster"), "Message"="test", "Message Data"=w179) -> (w181:T14)
        n116 = Enqueue Element(queue=w177, element=w181, error in (no error)=w176) -> ()  [unwired: 1 in, 3 out]
      }
    }
    n117 = case shown="1" w128 {
      tunnel: [w234 w235 w243] -> w136
      tunnel: w100 -> [_ w239 w245]
      tunnel: w99 -> [w234 w238 w244]
      tunnel: w132 -> [_ w237 _]
      frame 0, Default {
      }
      frame 2 {
        n118 = To Variant(anything=w237) -> (Variant=w241:variant)
        n119 = Bundle By Name(cluster=T14 {"Message"="", "Message Data"=variant} ("Message Cluster"), "Message"="WYSLIJ", "Message Data"=w241) -> (w242:T14)
        n120 = Enqueue Element(queue=w239, element=w242, error in (no error)=w238) -> (error out=w235:errorcluster)  [unwired: 1 in, 2 out]
      }
      frame 1 {
        n121 = disable-structure shown="Disabled" {
          disable-tunnel: w245 -> [w249 _]
          disable-tunnel: w244 -> [w248 _]
          disable-tunnel: [w247 _] -> w243
          frame Disabled {
            n122 = for {
              N: 2 -> [_]
              tunnel: w249 -> [w253]
              shift-right: [w251] -> w247
              shift-left: w248 -> [w252]
              n123 = call "send queue.vi"("zerowanie predkosci"=T4[] [{"identifier"=1, "extended?"=FALSE, "type"=0, "payload"=[1, 0, 0, 0, 0, 0, 0, 0]}, {"identifier"=2, "extended?"=FALSE, "type"=0, "payload"=[0, 0, 0, 0, 0, 0, 0]}], "error in (no error)"=w252, "Queue in"=w253) -> ("error out"=w251:errorcluster)  [unwired: 7 in, 1 out]
            }
          }
          frame Enabled {
          }
        }
      }
    }
    n124 = shared-variable "NI-sbRIO9636-01A93195\\FPGA.lvlib\\Elapsed Time (s)"() -> (w87:dbl)  [unwired: 1 in, 1 out]
    n125 = local read "timestamp last"() -> (w90:timestamp)
    n126 = Greater?(x=w87, y=w89) -> (0:w88:bool)
    n127 = case shown="True" w88 {
      frame False {
      }
      frame True {
        n128 = property on="Przestarzała data" class="Bool (strict)"("Colors [4]"=cluster{u32, u32}[] [{16751378, 16751378}, {14420480, 16720896}]) -> ()  [unwired: 2 in, 2 out]
      }
    }
    n129 = Subtract(x=w97, y=w90) -> (x-y=w94:dbl)
    "tim 2" <- w94
    n130 = call <vilib>:"Mean PtByPt.vi"("x"=w94, "sample length"=w93) -> ("mean"=w95:dbl)  [unwired: 2 in, 1 out]
    n131 = Bundle("mean"=w95) -> (→"Waveform Chart":cluster{"mean":dbl})  [unwired: 1 in]
  }
  n132 = while {
    tunnel: w13 -> [w294]
    tunnel: w12 -> [w293]
    tunnel: [w291] -> w16
    i -> [w292]
    stop <- "stop UDP 2" stop-if-true
    n133 = case shown="True" "UDP to sb 2" {
      tunnel: w294 -> [_ w310]
      tunnel: w293 -> [w297 w309]
      tunnel: [w297 w306] -> w291
      frame False {
      }
      frame True {
        w300 = u16 58431  # port
        w303 = u16 58432  # remote port
        w301 = "192.168.1.101"  # address
        w312 = 56 items=["No Error", "Argument Error", "Memory Full", "Out of Zone", "End of File", "File Already Open", "Generic File IO Error", "File Not Found", "File Permission Error", "Disk Full", "Duplicate Path", "Too Many Files Open", "Not Enabled", "Resource File Not Found", "Cannot Add Resource", "Resource Not Found", "Image Not Found", "Image Memory Error", "Pen Does Not Exist", "Config Bad Type", "Config Token Not Found", "Config Parse Error", "Config Memory Error", "Bad External Code Format", "Bad External Code Offset", "External Code Not Present", "Null Window", "Destroy Window Mixup", "Null Menu", "Print Aborted", "Bad Print Record", "Print Driver Error", "Windows Error During Print", "Memory Error During Print", "Print Dialog Error", "Generic Print Error", "Invalid Device Refnum", "Device Not Found", "Device Parameter Error", "Device Unit Error", "Can't Open Device", "Device Call Aborted", "Generic Error", "Cancelled By User", "Object ID Too Low", "Object ID Too High", "Object Not In Heap", "Unknown Heap", "Bad DefProc ID", "DefProc Not In Table", "Message Out Of Range", "Null Method", "Unknown Message", "Manager Call Not Supported", "Bad address", "Connection In progress", "Connection timed out", "Connection is already in progress", "Network attribute not supported", "Network error", "Address in use", "System out of memory", "Connection aborted", "Connection refused", "Connection is not connected", "Connection is already connected", "Connection closed", "Initialize error (interapplication manager)", "Bad occurrence", "Wait on unbound occurrence handler", "Occurrence queue overflow", "Bad path", "Semaphore not signaled", "Unrecognized type (interapplication manager)"] ("3rd Error to Convert")
        w313 = 62 items=["No Error", "Argument Error", "Memory Full", "Out of Zone", "End of File", "File Already Open", "Generic File IO Error", "File Not Found", "File Permission Error", "Disk Full", "Duplicate Path", "Too Many Files Open", "Not Enabled", "Resource File Not Found", "Cannot Add Resource", "Resource Not Found", "Image Not Found", "Image Memory Error", "Pen Does Not Exist", "Config Bad Type", "Config Token Not Found", "Config Parse Error", "Config Memory Error", "Bad External Code Format", "Bad External Code Offset", "External Code Not Present", "Null Window", "Destroy Window Mixup", "Null Menu", "Print Aborted", "Bad Print Record", "Print Driver Error", "Windows Error During Print", "Memory Error During Print", "Print Dialog Error", "Generic Print Error", "Invalid Device Refnum", "Device Not Found", "Device Parameter Error", "Device Unit Error", "Can't Open Device", "Device Call Aborted", "Generic Error", "Cancelled By User", "Object ID Too Low", "Object ID Too High", "Object Not In Heap", "Unknown Heap", "Bad DefProc ID", "DefProc Not In Table", "Message Out Of Range", "Null Method", "Unknown Message", "Manager Call Not Supported", "Bad address", "Connection In progress", "Connection timed out", "Connection is already in progress", "Network attribute not supported", "Network error", "Address in use", "System out of memory", "Connection aborted", "Connection refused", "Connection is not connected", "Connection is already connected", "Connection closed", "Initialize error (interapplication manager)", "Bad occurrence", "Wait on unbound occurrence handler", "Occurrence queue overflow", "Bad path", "Semaphore not signaled", "Unrecognized type (interapplication manager)"] ("1st Error to Convert")
        n134 = String To IP(1:w301) -> (0:w302:u32)
        n135 = UDP Open(11:w300) -> (port=w299:refnum<k16>, 0:w298:errorcluster)  [unwired: 4 in, 1 out]
        n136 = Bundle("remote port"=w303, w302, "port"=w299, "error out"=w298) -> (w305:T19)  [unwired: 1 in]
        n137 = while {
          tunnel: [w325] -> w315
          tunnel: [w327] -> w304
          tunnel: w310 -> [w317]
          tunnel: w309 -> [w318]
          tunnel: [w324] -> w308
          tunnel: [w321] -> w307
          tunnel: w305 -> [w316]
          i -> [w323]
          stop <- w322 stop-if-true
          # "Wysylanie  do SBRIO"
          n138 = Wait (ms)(milliseconds to wait=u32 10) -> ()  [unwired: 1 out]
          n139 = call "Wysylanie UDP do SbRIO.vi"("Cluster"=w316, "error in queue"=w318, "queue in"=w317) -> ("error out queue"=w321:errorcluster, "error out udp"=w325:errorcluster, "queue out 2"=w324:refnum<queue>, "connection ID out"=w327:refnum<k16>, "stop error ?"=w320:bool)  [unwired: 4 in]
          n140 = Compound Arithmetic op=OR(w320, "udp to sbrio  2") -> (w322:bool)
          "send ind" <- w323
        }
        n141 = UDP Close(connection ID=w304, 8:w315) -> (error out=w314:errorcluster)  [unwired: 1 out]
        n142 = Release Queue(queue=w308, error in (no error)=w307) -> (error out=w306:errorcluster)  [unwired: 1 in, 2 out]
        n143 = call <vilib>:"Error to Warning.vi"("1st Error to Convert"=w313, "3rd Error to Convert"=w312, "error in"=w314) -> ("warning out"=w311:errorcluster)  [unwired: 3 in, 9 out]
        n144 = call <vilib>:"Simple Error Handler.vi"("error in (no error)"=w311) -> ()  [unwired: 1 in, 8 out]
      }
    }
    n145 = Wait Until Next ms Multiple(millisecond multiple=u32 1000 ("milliseconds to wait")) -> ()  [unwired: 1 out]
    "Numeric 3" <- w292
  }
  n146 = disable-structure shown="Disabled" {
    frame Disabled {
      n147 = while {
        stop <- "stop UDP" stop-if-true
        n148 = case shown="True" "UDP to sb" {
          frame False {
          }
          frame True {
            w357 = u16 58432  # remote port
            w361 = "192.168.1.100"  # address
            w365 = 56 items=["No Error", "Argument Error", "Memory Full", "Out of Zone", "End of File", "File Already Open", "Generic File IO Error", "File Not Found", "File Permission Error", "Disk Full", "Duplicate Path", "Too Many Files Open", "Not Enabled", "Resource File Not Found", "Cannot Add Resource", "Resource Not Found", "Image Not Found", "Image Memory Error", "Pen Does Not Exist", "Config Bad Type", "Config Token Not Found", "Config Parse Error", "Config Memory Error", "Bad External Code Format", "Bad External Code Offset", "External Code Not Present", "Null Window", "Destroy Window Mixup", "Null Menu", "Print Aborted", "Bad Print Record", "Print Driver Error", "Windows Error During Print", "Memory Error During Print", "Print Dialog Error", "Generic Print Error", "Invalid Device Refnum", "Device Not Found", "Device Parameter Error", "Device Unit Error", "Can't Open Device", "Device Call Aborted", "Generic Error", "Cancelled By User", "Object ID Too Low", "Object ID Too High", "Object Not In Heap", "Unknown Heap", "Bad DefProc ID", "DefProc Not In Table", "Message Out Of Range", "Null Method", "Unknown Message", "Manager Call Not Supported", "Bad address", "Connection In progress", "Connection timed out", "Connection is already in progress", "Network attribute not supported", "Network error", "Address in use", "System out of memory", "Connection aborted", "Connection refused", "Connection is not connected", "Connection is already connected", "Connection closed", "Initialize error (interapplication manager)", "Bad occurrence", "Wait on unbound occurrence handler", "Occurrence queue overflow", "Bad path", "Semaphore not signaled", "Unrecognized type (interapplication manager)"] ("3rd Error to Convert")
            w366 = 62 items=["No Error", "Argument Error", "Memory Full", "Out of Zone", "End of File", "File Already Open", "Generic File IO Error", "File Not Found", "File Permission Error", "Disk Full", "Duplicate Path", "Too Many Files Open", "Not Enabled", "Resource File Not Found", "Cannot Add Resource", "Resource Not Found", "Image Not Found", "Image Memory Error", "Pen Does Not Exist", "Config Bad Type", "Config Token Not Found", "Config Parse Error", "Config Memory Error", "Bad External Code Format", "Bad External Code Offset", "External Code Not Present", "Null Window", "Destroy Window Mixup", "Null Menu", "Print Aborted", "Bad Print Record", "Print Driver Error", "Windows Error During Print", "Memory Error During Print", "Print Dialog Error", "Generic Print Error", "Invalid Device Refnum", "Device Not Found", "Device Parameter Error", "Device Unit Error", "Can't Open Device", "Device Call Aborted", "Generic Error", "Cancelled By User", "Object ID Too Low", "Object ID Too High", "Object Not In Heap", "Unknown Heap", "Bad DefProc ID", "DefProc Not In Table", "Message Out Of Range", "Null Method", "Unknown Message", "Manager Call Not Supported", "Bad address", "Connection In progress", "Connection timed out", "Connection is already in progress", "Network attribute not supported", "Network error", "Address in use", "System out of memory", "Connection aborted", "Connection refused", "Connection is not connected", "Connection is already connected", "Connection closed", "Initialize error (interapplication manager)", "Bad occurrence", "Wait on unbound occurrence handler", "Occurrence queue overflow", "Bad path", "Semaphore not signaled", "Unrecognized type (interapplication manager)"] ("1st Error to Convert")
            n149 = UDP Open(11:u16 58431 ("port")) -> (port=w360:refnum<k16>, 0:w359:errorcluster)  [unwired: 4 in, 1 out]
            n150 = String To IP(1:w361) -> (0:w358:u32)
            n151 = while {
              tunnel: w360 -> [w374]
              tunnel: w359 -> [w373]
              tunnel: [w383] -> w368
              tunnel: [w384] -> w363
              tunnel: w358 -> [w376]
              tunnel: w357 -> [w375]
              i -> [w372]
              stop <- w381 stop-if-true
              # "tutaj dodaje sie zmienne lokalne \ndo clustera jakie chces zwyslac"
              # "Wysylanie  do SBRIO"
              n152 = local read "cluster manipulator"() -> (w369:T12)
              n153 = local read "cluster jazda"() -> (w370:T13)
              n154 = Bundle By Name(cluster=T20 {"cluster_jazda"={"pwmjazda"=0.0, "skretjazda"=0.0, "obrotjazda"=0.0, "hamowaniejazda"=0.0}, "cluster_manipulator"={"pwm 1"=0.0, "pwm 2"=0.0, "pwm 3"=0.0, "pwm 4"=0.0, "pwm 5"=0.0, "pwm 6"=0.0, "pwm 7"=0.0}, "GIMBALE"={"Gimbal 1"={"OSY"=0.0, "OSY X"=0.0}, "Gimbal 2"={"OSY"=0.0, "OSY X"=0.0}}} ("output cluster"), "cluster_jazda"=w370, "cluster_manipulator"=w369) -> (w378:T20)
              n155 = Type Cast(x=w378) -> (*(type *) &x=w377:string)  [unwired: 1 out]
              n156 = UDP Write(address=w376, port or service name=w375, connection ID=w374, data in=w377, 8:w373) -> (error out=w383:errorcluster, 3:w384:refnum<k16>)  [unwired: 1 in]
              n157 = Wait (ms)(milliseconds to wait=u32 10) -> ()  [unwired: 1 out]
              n158 = Unbundle By Name(w383) -> ("status"=w382:bool)
              n159 = Or(x=w382, y="udp to sbrio") -> (x .or. y?=w381:bool)
              "Numeric" <- w372
            }
            n160 = UDP Close(connection ID=w363, 8:w368) -> (error out=w367:errorcluster)  [unwired: 1 out]
            n161 = call <vilib>:"Error to Warning.vi"("1st Error to Convert"=w366, "3rd Error to Convert"=w365, "error in"=w367) -> ("warning out"=w364:errorcluster)  [unwired: 3 in, 9 out]
            n162 = call <vilib>:"Simple Error Handler.vi"("error in (no error)"=w364) -> ()  [unwired: 1 in, 8 out]
          }
        }
      }
      n163 = while {
        stop <- w328 stop-if-true
        n164 = case shown="True" "UDP from sb" {
          frame False {
          }
          frame True {
            w333 = 56 items=["No Error", "Argument Error", "Memory Full", "Out of Zone", "End of File", "File Already Open", "Generic File IO Error", "File Not Found", "File Permission Error", "Disk Full", "Duplicate Path", "Too Many Files Open", "Not Enabled", "Resource File Not Found", "Cannot Add Resource", "Resource Not Found", "Image Not Found", "Image Memory Error", "Pen Does Not Exist", "Config Bad Type", "Config Token Not Found", "Config Parse Error", "Config Memory Error", "Bad External Code Format", "Bad External Code Offset", "External Code Not Present", "Null Window", "Destroy Window Mixup", "Null Menu", "Print Aborted", "Bad Print Record", "Print Driver Error", "Windows Error During Print", "Memory Error During Print", "Print Dialog Error", "Generic Print Error", "Invalid Device Refnum", "Device Not Found", "Device Parameter Error", "Device Unit Error", "Can't Open Device", "Device Call Aborted", "Generic Error", "Cancelled By User", "Object ID Too Low", "Object ID Too High", "Object Not In Heap", "Unknown Heap", "Bad DefProc ID", "DefProc Not In Table", "Message Out Of Range", "Null Method", "Unknown Message", "Manager Call Not Supported", "Bad address", "Connection In progress", "Connection timed out", "Connection is already in progress", "Network attribute not supported", "Network error", "Address in use", "System out of memory", "Connection aborted", "Connection refused", "Connection is not connected", "Connection is already connected", "Connection closed", "Initialize error (interapplication manager)", "Bad occurrence", "Wait on unbound occurrence handler", "Occurrence queue overflow", "Bad path", "Semaphore not signaled", "Unrecognized type (interapplication manager)"] ("3rd Error to Convert")
            w332 = 62 items=["No Error", "Argument Error", "Memory Full", "Out of Zone", "End of File", "File Already Open", "Generic File IO Error", "File Not Found", "File Permission Error", "Disk Full", "Duplicate Path", "Too Many Files Open", "Not Enabled", "Resource File Not Found", "Cannot Add Resource", "Resource Not Found", "Image Not Found", "Image Memory Error", "Pen Does Not Exist", "Config Bad Type", "Config Token Not Found", "Config Parse Error", "Config Memory Error", "Bad External Code Format", "Bad External Code Offset", "External Code Not Present", "Null Window", "Destroy Window Mixup", "Null Menu", "Print Aborted", "Bad Print Record", "Print Driver Error", "Windows Error During Print", "Memory Error During Print", "Print Dialog Error", "Generic Print Error", "Invalid Device Refnum", "Device Not Found", "Device Parameter Error", "Device Unit Error", "Can't Open Device", "Device Call Aborted", "Generic Error", "Cancelled By User", "Object ID Too Low", "Object ID Too High", "Object Not In Heap", "Unknown Heap", "Bad DefProc ID", "DefProc Not In Table", "Message Out Of Range", "Null Method", "Unknown Message", "Manager Call Not Supported", "Bad address", "Connection In progress", "Connection timed out", "Connection is already in progress", "Network attribute not supported", "Network error", "Address in use", "System out of memory", "Connection aborted", "Connection refused", "Connection is not connected", "Connection is already connected", "Connection closed", "Initialize error (interapplication manager)", "Bad occurrence", "Wait on unbound occurrence handler", "Occurrence queue overflow", "Bad path", "Semaphore not signaled", "Unrecognized type (interapplication manager)"] ("1st Error to Convert")
            n165 = UDP Open(9:1000 ("timeout ms (25000)"), 11:u16 61558 ("port")) -> (port=w338:refnum<k16>, 0:w337:errorcluster)  [unwired: 3 in, 1 out]
            n166 = while {
              tunnel: w338 -> [w345]
              tunnel: w337 -> [w344]
              tunnel: [w353] -> w336
              tunnel: [w349] -> w335
              i -> [w347]
              stop <- "UDP odbior" stop-if-true
              # "Odiór satusu z SBRIO"
              n167 = UDP Read(connection ID=w345, max size (548)=4, timeout ms (25000)=5000, 8:w344) -> (data out=w354:string, error out=w349:errorcluster, 3:w353:refnum<k16>)  [unwired: 2 out]
              n168 = Unbundle By Name(w349) -> ("status"=→"brak polaczenia":bool)
              n169 = Type Cast(type=u16 0, x=w354) -> (*(type *) &x=w342:u16)
              n170 = Number To Boolean Array(number=w342) -> (Boolean array=w352:bool[])
              n171 = Index Array(array=w352, index=0) -> (element=→"połączenie RT":bool)
              "Numeric 2" <- w347
            }
            n172 = UDP Close(connection ID=w336, 8:w335) -> (error out=w331:errorcluster)  [unwired: 1 out]
            n173 = call <vilib>:"Error to Warning.vi"("1st Error to Convert"=w332, "3rd Error to Convert"=w333, "error in"=w331) -> ("warning out"=w334:errorcluster)  [unwired: 3 in, 9 out]
            n174 = call <vilib>:"Simple Error Handler.vi"("error in (no error)"=w334) -> ()  [unwired: 1 in, 8 out]
          }
        }
        n175 = local read "stop UDP"() -> (w328:bool)
      }
    }
    frame Enabled {
    }
  }
  n176 = while {
    tunnel: [w418] -> w22
    tunnel: [w417] -> w21
    tunnel: w13 -> [w393]
    tunnel: w12 -> [w392]
    tunnel: [w391] -> w11
    stop <- w387 stop-if-true
    # "SPRAWDZ BEZ CASE SAM DELAY"
    # "Manipulator"
    n177 = local read "stop all"() -> (w387:bool)
    n178 = Wait (ms)(milliseconds to wait=u32 10) -> ()  [unwired: 1 out]
    n179 = control-ref of="wysylanie"() -> (w429:refnum<vi>)
    n180 = call "Optim joy manipulator.vi"("device index"="device index") -> ("error out"=w417:errorcluster, "POV"=w404:bool, "Refnum out"=w418:refnum<k1>, "Cluster"=w402:T21, "wysylanie"=w406:bool, "axis info"=w397:T5)  [unwired: 5 in]
    "wysylanie" <- w406
    n181 = Unbundle(w397) -> ("X axis"=w416:i32, "Y axis"=w430:i32, "Z axis"=w421:i32, "X axis rotation"=w395:i32, "Y axis rotation"=w394:i32)  [unwired: 3 out]
    n182 = call "blokada wysylania manipulatora.vi"("Y"=w430, "Zaxis"=w421, "X axis"=w416, "Boolean in"=w429) -> ("zakres Z"=→"zakres Z":bool, "zakres X"=→"zakres X":bool, "blokadaa"=→"blokadaa":bool, "zakres Y"=→"zakres Y":bool)  [unwired: 4 in]
    n183 = call "osie na grafie.vi"("Y axis rotation"=w394, "X axis rotation"=w395, "X axis"=w416, "Y axis"=w430) -> ("graph 2"=→"graph 2":cluster{i32[], i32[]}[])  [unwired: 7 in]
    n184 = feedback-in #2(w406) -> ()
    n185 = feedback #2() -> (w434:bool)  [unwired: 1 in]
    n186 = Unbundle(w402) -> ("button 1"=w399:bool, "button 2"=w398:bool, "button 3"=→"button 3":bool, "button 4"=→"button 4":bool)  [unwired: 1 out]
    "button 1" <- w399
    "button 2" <- w398
    n187 = case shown="True" TRUE {
      tunnel: [w447 w450] -> w405
      tunnel: w434 -> [w446 w449]
      tunnel: w406 -> [w445 w448]
      frame True {
        n188 = And(x=w445, y=w446) -> (x .and. y?=w447:bool)
      }
      frame False {
        n189 = And(x=w448, y=w449) -> (x .and. y?=w450:bool)
      }
    }
    n190 = call "Simple Edge Detection.vi"("Mode"=T16."Falling Edge", "clk_in"=w405) -> ("edge?"=w408:bool)  [unwired: 9 in]
    n191 = call "Manipulator PWM-y.vi"("Boolean"=w404, "button in"=w398, "X axis"=w416, "button 1"=w399, "Z axis"=w421, "Y"=w430) -> ("String"=w403:string)  [unwired: 5 in]
    "String wysylany" <- w403
    n192 = Or(x=w405, y=w408) -> (x .or. y?=w432:bool)
    n193 = local read "blokadaa"() -> (w407:bool)
    n194 = Not(x=w407) -> (.not. x?=w431:bool)
    n195 = Scan From String(format string="%d %d %d %d %d %d %d", input string="Strin wysłany") -> (output 1=w415:dbl, output 2=w414:dbl, output 3=w413:dbl, output 4=w412:dbl, output 5=w411:dbl, output 6=w410:dbl, output 7=w409:dbl)  [unwired: 9 in, 3 out]
    "pwm 1" <- w415
    "pwm 2" <- w414
    "pwm 3" <- w413
    "pwm 4" <- w412
    "pwm 5" <- w411
    "pwm 6" <- w410
    "pwm 7" <- w409
    n196 = And(x=w432, y=w431) -> (x .and. y?=w388:bool)
    n197 = case shown="True" w388 {
      tunnel: w403 -> [_ w451]
      frame False {
      }
      frame True {
        n198 = local write "Strin wysłany"(w451) -> ()
      }
    }
    n199 = Bundle By Name(cluster=T12 {"pwm 1"=0.0, "pwm 2"=0.0, "pwm 3"=0.0, "pwm 4"=0.0, "pwm 5"=0.0, "pwm 6"=0.0, "pwm 7"=0.0} ("output cluster"), "pwm 1"=w415, "pwm 2"=w414, "pwm 3"=w413, "pwm 4"=w412, "pwm 5"=w411, "pwm 6"=w410, "pwm 7"=w409) -> (w390:T12)
    "cluster manipulator" <- w390
    n200 = call "PWM to CAN.vi"("cluster manipulator 2"=w390, "serwa i pompa"="serwa i pompa", "MANIPULATOR ID 3"="MANIPULATOR ID 3") -> ("array of cans"=w389:T4[])  [unwired: 6 in, 2 out]
    n201 = case shown="True" w388 {
      tunnel: w393 -> [_ w441]
      tunnel: w392 -> [w436 w440]
      tunnel: [w436 w438] -> w391
      tunnel: w389 -> [_ w437]
      frame False {
      }
      frame True {
        n202 = To Variant(anything=w437) -> (Variant=w442:variant)
        n203 = Bundle By Name(cluster=T14 {"Message"="", "Message Data"=variant} ("Message Cluster"), "Message"="WYSLIJ", "Message Data"=w442) -> (w439:T14)
        n204 = Enqueue Element(queue=w441, element=w439, error in (no error)=w440) -> (error out=w438:errorcluster)  [unwired: 1 in, 2 out]
      }
    }
  }
  n205 = disable-structure shown="Disabled" {
    frame Disabled {
      n206 = while {
        stop <- w452 stop-if-true
        n207 = case shown="True" "ON/OFF CAM" {
          frame False {
          }
          frame True {
            n208 = call "IMAQ Create"("Image Name"="Grab and Reconfigure") -> ("New Image"=w454:T11)  [unwired: 3 in, 2 out]
            n209 = while {
              shift-right: [w469] -> w460
              shift-left: _ -> [w466]
              shift-right: [w465] -> w459
              shift-left: errorcluster {"status"=FALSE, "code"=0, "source"=""} ("error out") -> [w473]
              tunnel: w454 -> [w464]
              stop <- w475 stop-if-true
              n210 = Not A Number/Path/Refnum?(number/path/refnum=w466) -> (NaN/Path/Refnum?=w467:bool)
              n211 = case shown="True" w467 {
                tunnel: w466 -> [w486 _]
                tunnel: [w486 w491] -> w474
                tunnel: w473 -> [w485 _]
                tunnel: [w485 w490] -> w472
                tunnel: "Camera Name" -> [_ w488]
                frame False {
                }
                frame True {
                  n212 = call <vilib>:"IMAQdx Open Camera.vi"("Session In"=w488) -> ("error out"=w492:errorcluster, "Session Out"=w493:T22)  [unwired: 2 in, 7 out]
                  n213 = call <vilib>:"IMAQdx Configure Grab.vi"("error in"=w492, "Session In"=w493) -> ("error out"=w490:errorcluster, "Session Out"=w491:T22)  [unwired: 8 out]
                  n214 = Unbundle By Name(w490) -> ("status"=w489:bool)
                  n215 = Not(x=w489) -> (.not. x?=→"Acquiring":bool)
                }
              }
              n216 = call <vilib>:"IMAQdx Grab2.vi"("error in"=w472, "Image In"=w464, "Session In"=w474) -> ("error out"=w471:errorcluster, "Buffer Number Out"=→"Buffer Number 3":u32, "Image Out"=→"Image":T11, "Session Out"=w470:T22)  [unwired: 5 in]
              n217 = case shown="Error" w471 {
                selector: w471 -> [w477 w481]
                tunnel: [w477 errorcluster {"status"=FALSE, "code"=0, "source"=""} ("error IO")] -> w465
                tunnel: w470 -> [w476 w482]
                tunnel: [w476 w479] -> w469
                tunnel: "Camera Name" -> [_ w479]
                frame No Error {
                }
                frame Error {
                  n218 = call <vilib>:"IMAQdx Close Camera.vi"("error in"=w481, "Session In"=w482) -> ("error out"=w480:errorcluster)  [unwired: 9 out]
                  n219 = call <vilib>:"Clear Errors.vi"("error in (no error)"=w480) -> ()  [unwired: 5 in, 2 out]
                  n220 = local write "Acquiring"(FALSE ("Acquiring")) -> ()
                  n221 = Wait (ms)(milliseconds to wait=u32 250) -> ()  [unwired: 1 out]
                }
              }
              n222 = Or(x=w465, y="Stop 2") -> (x .or. y?=w475:bool)
            }
            n223 = call <vilib>:"IMAQdx Close Camera.vi"("error in"=w459, "Session In"=w460) -> ("error out"=w456:errorcluster)  [unwired: 9 out]
            n224 = call "Imaq Dispose"("Image"=w454, "error in (no error)"=w456) -> ("error out"=w455:errorcluster)  [unwired: 4 in]
            n225 = call <vilib>:"General Error Handler.vi"("error in (no error)"=w455) -> ()  [unwired: 2 in, 13 out]
          }
        }
        n226 = local read "stop UDP"() -> (w452:bool)
      }
    }
    frame Enabled {
    }
  }
  n227 = while {
    shift-right: [w498] -> _
    shift-left: w5 -> [w532]
    tunnel: w3 -> [w528]
    tunnel: w2 -> [w527]
    i -> [w499]
    stop <- w520 stop-if-true
    w535 = u32 5  # milliseconds to wait
    # "odczyt CANA"
    n228 = Get Queue Status(queue=w528, error in (no error)=w527) -> (queue out=w526:refnum<queue>, error out=w525:errorcluster, # elements in queue=→"kolejka odbior":i32)  [unwired: 1 in, 5 out]
    n229 = Dequeue Element(queue=w526, error in (no error)=w525) -> (element=w531:T14)  [unwired: 1 in, 3 out]
    n230 = Unbundle By Name(w531) -> ("Message Data"=w530:variant)
    n231 = Wait (ms)(milliseconds to wait=w535) -> ()  [unwired: 1 out]
    n232 = local read "stop all"() -> (w520:bool)
    n233 = Variant To Data(type=T4 {"identifier"=0, "extended?"=FALSE, "type"=0, "payload"=[]} ("CAN frame 3"), Variant=w530) -> (data=w523:T4)  [unwired: 1 in, 1 out]
    n234 = Unbundle By Name(w523) -> ("payload"=w522:u8[])
    n235 = Empty Array?(array=w522) -> (empty?=w521:bool)
    n236 = feedback #3() -> (w497:u16)  [unwired: 1 in]
    n237 = feedback #4() -> (w494:string)  [unwired: 1 in]
    "wilgotność i temperatura" <- w494
    n238 = case shown="False" w521 {
      tunnel: "Widocznosc ramek" -> [w545 _]
      tunnel: [w544 w550] -> w498
      tunnel: w532 -> [w543 w550]
      tunnel: "Hexadecimal?" -> [w542 _]
      tunnel: w523 -> [w538 _]
      tunnel: [w537 w549] -> w496
      tunnel: w497 -> [_ w549]
      tunnel: [w536 w548] -> w495
      tunnel: w494 -> [_ w548]
      frame False {
        w539 = 0.0  # Numeric
        n239 = Get Date/Time In Seconds() -> (seconds since 1Jan1904=w546:timestamp)
        n240 = feedback #5(w539) -> (w540:dbl)
        n241 = call "NI-Embedded CAN for RIO subVI - CAN Frame to Table test.vi"("Boolean"=w545, "Hexadecimal?"=w542, "x"=w540, "timestamp"=w546, "Input Array"=w543, "CAN frame"=w538) -> ("Numeric"=w541:dbl, "(hi.lo)"=w537:u16, "string"=w536:string, "Output Array"=w544:string[][], "okres 100"=→"okres 100[ms]":dbl)  [unwired: 1 in]
        "ilosc mesagy" <- w541
        n242 = feedback-in #5(w541) -> ()
      }
      frame True {
      }
    }
    "Frames" <- w498
    "PH" <- w496
    n243 = feedback-in #3(w496) -> ()
    n244 = feedback-in #4(w495) -> ()
    n245 = call "telemetria.vi"("Output Array"=w498) -> ("średnie"=w519:T6, "raw"=w518:cluster{u16, u16, u16, u16, u16, u16})  [unwired: 3 in, 6 out]
    "wszystkie" <- w519
    n246 = Unbundle(w518) -> (w506:u16, w507:u16, w508:u16, w509:u16, w510:u16, w511:u16)
    n247 = Unbundle(w519) -> ("mean"=w517:dbl, "mean"=w516:dbl, "mean"=w515:dbl, "mean"=w514:dbl, "mean"=w513:dbl, "mean"=w512:dbl)
    n248 = Bundle("mean"=w514, w509) -> (→"PRZOD L":cluster{"mean":dbl, u16})  [unwired: 1 in]
    n249 = Bundle("mean"=w513, w510) -> (→"TYL L":cluster{"mean":dbl, u16})  [unwired: 1 in]
    n250 = Bundle("mean"=w512, w511) -> (→"SRODEK L":cluster{"mean":dbl, u16})  [unwired: 1 in]
    n251 = Bundle("mean"=w517, w506) -> (→"przod P":cluster{"mean":dbl, u16})  [unwired: 1 in]
    n252 = Bundle("mean"=w515, w508) -> (→"Środek P":cluster{"mean":dbl, u16})  [unwired: 1 in]
    n253 = Bundle("mean"=w516, w507) -> (→"Tyl P":cluster{"mean":dbl, u16})  [unwired: 1 in]
    "Numeric 5" <- w499
  }
  n254 = while {
    tunnel: w13 -> [w554]
    tunnel: w12 -> [w553]
    tunnel: [w551] -> w15
    i -> [w552]
    stop <- w555 stop-if-true
    # "config"
    n255 = event shown="[8] \"PRZOD L.OK Button\": Value Change" {
      selector: _ -> [_ _ _ _ _ _ _ _ _ _ _]
      dyn-events: _ -> [_ _ _ _ _ _ _ _ _ _ _]
      timeout: _ -> [_ _ _ _ _ _ _ _ _ _ _]
      tunnel: [_ TRUE _ _ _ _ _ _ _ _ _] -> w555
      tunnel: w554 -> [_ _ w560 w564 _ w566 w570 w590 w597 w601 w605]
      tunnel: w553 -> [_ _ w559 w563 _ w567 w571 w591 w596 w600 w604]
      tunnel: [_ _ w557 _ _ _ _ _ _ _ _] -> w551
      event Timeout {
        n256 = event-data() -> ()  [unwired: 1 in, 3 out]
      }
      event "eventy stop": Value Change {
        n257 = event-data() -> ()  [unwired: 1 in, 6 out]
      }
      event "stop queue": Value Change {
        n258 = event-data() -> ()  [unwired: 1 in, 6 out]
        n259 = Enqueue Element(queue=w560, element=T14 {"Message"="Exit", "Message Data"=variant}, error in (no error)=w559) -> (error out=w557:errorcluster)  [unwired: 1 in, 2 out]
      }
      event Value Change {
        n260 = event-data() -> ()  [unwired: 1 in, 6 out]
        n261 = call "PrzódL.vi"("Konfiguracja"="PRZOD P") -> ("Message Cluster"=w562:T14)  [unwired: 10 in]
        n262 = Enqueue Element(queue=w564, element=w562, error in (no error)=w563) -> ()  [unwired: 1 in, 3 out]
      }
      event "E-Stop": Value Change {
        n263 = event-data() -> ()  [unwired: 1 in, 6 out]
      }
      event Value Change {
        n264 = event-data() -> ()  [unwired: 1 in, 6 out]
        n265 = call "PrzódL.vi"("Konfiguracja"="SRODEK P") -> ("Message Cluster"=w568:T14)  [unwired: 10 in]
        n266 = Enqueue Element(queue=w566, element=w568, error in (no error)=w567) -> ()  [unwired: 1 in, 3 out]
      }
      event Value Change {
        n267 = event-data() -> ()  [unwired: 1 in, 6 out]
        n268 = call "PrzódL.vi"("Konfiguracja"="TYL P") -> ("Message Cluster"=w572:T14)  [unwired: 10 in]
        n269 = Enqueue Element(queue=w570, element=w572, error in (no error)=w571) -> ()  [unwired: 1 in, 3 out]
      }
      event "Stop wózek", "Wózek up", "Wózek down", "Głębokość PWM", "Stop głębokość", "Wózek PWM", "Wiertło PWM", "ON/OFF Wiertło", "SERWO 4", "SERWO 5", "SERWO 6", "SERWO 3": Value Change {
        n270 = event-data() -> ()  [unwired: 1 in, 5 out]
        n271 = local read "PROBNK ID 4"() -> (w585:u32)
        n272 = Bundle("SERWO 6"="SERWO 6", "SERWO 5"="SERWO 5", "SERWO 4"="SERWO 4", "SERWO 3"="SERWO 3", "ON/OFF Wiertło"="ON/OFF Wiertło", "Wiertło PWM"="Wiertło PWM", "Wózek PWM"="Wózek PWM", "Stop głębokość"="Stop głębokość", "Głębokość PWM"="Głębokość PWM", "speed wózek"="speed wózek", "Wózek up"="Wózek up", "Wózek down"="Wózek down", "Stop wózek"="Stop wózek", "PROBNK ID 4"=w585) -> (w573:T23)  [unwired: 1 in]
        n273 = call "próbnik.vi"("output cluster 2"=w573) -> ("Message Cluster"=w584:T14, "number stopy"=w578:u32)  [unwired: 9 in]
        n274 = Enqueue Element(queue=w590, element=w584, error in (no error)=w591) -> ()  [unwired: 1 in, 3 out]
        n275 = case shown="4, 5" w578 {
          frame 2, 3 {
            n276 = property on="Wózek PWM" class="Slide (strict)"("Value"=u8 128 ("Wózek PWM")) -> ()  [unwired: 2 in, 2 out]
          }
          frame 0, Default {
            n277 = property on="Wiertło PWM" class="Slide (strict)"("Value"=u8 128 ("Wózek PWM")) -> ()  [unwired: 2 in, 2 out]
          }
          frame 1 {
          }
          frame 4, 5 {
            n278 = property on="Głębokość PWM" class="Slide (strict)"("Value"=u8 128 ("Wózek PWM")) -> ()  [unwired: 2 in, 2 out]
          }
        }
      }
      event Value Change {
        n279 = event-data() -> ()  [unwired: 1 in, 6 out]
        n280 = call "PrzódL.vi"("Konfiguracja"="PRZOD L") -> ("Message Cluster"=w598:T14)  [unwired: 10 in]
        n281 = Enqueue Element(queue=w597, element=w598, error in (no error)=w596) -> ()  [unwired: 1 in, 3 out]
      }
      event Value Change {
        n282 = event-data() -> ()  [unwired: 1 in, 6 out]
        n283 = call "PrzódL.vi"("Konfiguracja"="TYL L") -> ("Message Cluster"=w602:T14)  [unwired: 10 in]
        n284 = Enqueue Element(queue=w601, element=w602, error in (no error)=w600) -> ()  [unwired: 1 in, 3 out]
      }
      event Value Change {
        n285 = event-data() -> ()  [unwired: 1 in, 6 out]
        n286 = call "PrzódL.vi"("Konfiguracja"="SRODEK L") -> ("Message Cluster"=w606:T14)  [unwired: 10 in]
        n287 = Enqueue Element(queue=w605, element=w606, error in (no error)=w604) -> ()  [unwired: 1 in, 3 out]
      }
    }
    "eventy ind" <- w552
  }
  n288 = call <vilib>:"Simple Error Handler.vi"("error in (no error)"=w1) -> ()  [unwired: 1 in, 8 out]
  n289 = call-poly <vilib>:"Close Input Device.vi"("error in (no error)"=w21, "device ID"=w22) -> ("error out"=w20:errorcluster)  [unwired: 8 in]
  n290 = call <vilib>:"Simple Error Handler.vi"("error in (no error)"=w20) -> ()  [unwired: 1 in, 8 out]
  n291 = call-poly <vilib>:"Close Input Device.vi"("error in (no error)"=w23, "device ID"=w24) -> ("error out"=w19:errorcluster)  [unwired: 8 in]
  n292 = Merge Errors(w15, w14) -> (w10:errorcluster)
  n293 = call <vilib>:"Simple Error Handler.vi"("error in (no error)"=w19) -> ()  [unwired: 1 in, 8 out]
  n294 = Merge Errors(w10, w11) -> (w9:errorcluster)
  n295 = Merge Errors(w9, w16) -> (w17:errorcluster)
  n296 = call <vilib>:"Simple Error Handler.vi"("error in (no error)"=w17) -> ()  [unwired: 1 in, 8 out]
  n297 = disable-structure shown="Enabled" {
    frame Disabled {
      # "sterowanie kartezjańskie do manipulatora"
      n298 = call "ster kartezjan.vi"("Sterowanie w ukladzie narzędzia"="Sterowanie w ukladzie narzędzia") -> ("Digital in"=w617:refnum<vi>, "reference 2"=w616:refnum<vi>, "reference"=w615:refnum<vi>, "q1"=→"q1":dbl, "Py"=→"Py":dbl, "q2"=→"q2":dbl, "Pz"=→"Pz":dbl, "q3"=→"q3":dbl, "Px"=→"Px":dbl, "q4"=→"q4":dbl, "q5"=→"q5":dbl)  [unwired: 5 in, 3 out]
    }
    frame Enabled {
    }
  }
